vi "Autonomous Independent.vi"() -> ()   [LabVIEW 2016]
doc: "This VI is called when autonomous begins, and will automatically be terminated when autonomous ends. You can carry out timed or sensor driven robot movement independently without needing to return to the caller."
uses:
  <vilib>/Rock Robotics/WPI/Solenoid/WPI_SolenoidValue.ctl
  <vilib>/Rock Robotics/WPI/Utilities/WPI_GetSetVariantRefNum.vi
  <vilib>/addons/control/pid/pid.llb/PID (DBL).vi
  <vilib>/Rock Robotics/Network Tables/NT Write Number.vi
  <vilib>/Rock Robotics/WPI/RobotDrive/WPI_RobotDriveMecanumDrive_Cartesian.vi
  <vilib>/Rock Robotics/WPI/Solenoid/WPI_SolenoidSetEnum.vi
  <vilib>/addons/control/pid/NI_PID_pid.lvlib
panel:
  in  "PID gains 8":T1={"proportional gain (Kc)"=0.055, "integral time (Ti, min)"=0.0, "derivative time (Td, min)"=0.0} {"derivative time (Td, min)" format="%.3f"; "integral time (Ti, min)" format="%.3f"; "proportional gain (Kc)" format="%.3f"}
  out "Gauge 11":dbl(knob) scale=-180.0..180.0
  out "Gryo angle 11":dbl
  out "to motor 8":dbl
  in  "PID gains 12":T1={"proportional gain (Kc)"=0.055, "integral time (Ti, min)"=0.0, "derivative time (Td, min)"=0.0} {"derivative time (Td, min)" format="%.3f"; "integral time (Ti, min)" format="%.3f"; "proportional gain (Kc)" format="%.3f"}
  out "Gauge 15":dbl(knob) scale=-180.0..180.0
  out "Gryo angle 15":dbl
  out "to motor 12":dbl
  in  "PID gains 6":T1={"proportional gain (Kc)"=0.057, "integral time (Ti, min)"=0.0, "derivative time (Td, min)"=0.0} {"derivative time (Td, min)" format="%.3f"; "integral time (Ti, min)" format="%.3f"; "proportional gain (Kc)" format="%.3f"}
  out "Gauge 9":dbl(knob) scale=-180.0..180.0
  out "Gryo angle 9":dbl
  out "to motor 6":dbl
  in  "PID gains 7":T1={"proportional gain (Kc)"=0.055, "integral time (Ti, min)"=0.0, "derivative time (Td, min)"=0.0} {"derivative time (Td, min)" format="%.3f"; "integral time (Ti, min)" format="%.3f"; "proportional gain (Kc)" format="%.3f"}
  out "Gauge 10":dbl(knob) scale=-180.0..180.0
  out "Gryo angle 10":dbl
  out "to motor 7":dbl
  in  "PID gains 16":T1={"proportional gain (Kc)"=0.057, "integral time (Ti, min)"=0.0, "derivative time (Td, min)"=0.0} {"derivative time (Td, min)" format="%.3f"; "integral time (Ti, min)" format="%.3f"; "proportional gain (Kc)" format="%.3f"}
  out "Gauge 19":dbl(knob) scale=-180.0..180.0
  out "Gryo angle 19":dbl
  out "to motor 16":dbl
  in  "PID gains 19":T1={"proportional gain (Kc)"=0.057, "integral time (Ti, min)"=0.0, "derivative time (Td, min)"=0.0} {"derivative time (Td, min)" format="%.3f"; "integral time (Ti, min)" format="%.3f"; "proportional gain (Kc)" format="%.3f"}
  out "Gauge 26":dbl(knob) scale=-180.0..180.0
  out "Gryo angle 26":dbl
  out "to motor 23":dbl
  in  "PID gains 21":T1={"proportional gain (Kc)"=0.057, "integral time (Ti, min)"=0.0, "derivative time (Td, min)"=0.0} {"derivative time (Td, min)" format="%.3f"; "integral time (Ti, min)" format="%.3f"; "proportional gain (Kc)" format="%.3f"}
  out "Gauge 28":dbl(knob) scale=-180.0..180.0
  out "Gryo angle 28":dbl
  out "to motor 25":dbl
  in  "PID gains 48":T1={"proportional gain (Kc)"=0.057, "integral time (Ti, min)"=0.0, "derivative time (Td, min)"=0.0} {"derivative time (Td, min)" format="%.3f"; "integral time (Ti, min)" format="%.3f"; "proportional gain (Kc)" format="%.3f"}
  out "Gauge 55":dbl(knob) scale=-180.0..180.0
  out "Gryo angle 55":dbl
  out "to motor 52":dbl
  in  "PID gains 47":T1={"proportional gain (Kc)"=0.057, "integral time (Ti, min)"=0.0, "derivative time (Td, min)"=0.0} {"derivative time (Td, min)" format="%.3f"; "integral time (Ti, min)" format="%.3f"; "proportional gain (Kc)" format="%.3f"}
  out "Gauge 54":dbl(knob) scale=-180.0..180.0
  out "Gryo angle 54":dbl
  out "to motor 51":dbl
  in  "PID gains 46":T1={"proportional gain (Kc)"=0.057, "integral time (Ti, min)"=0.0, "derivative time (Td, min)"=0.0} {"derivative time (Td, min)" format="%.3f"; "integral time (Ti, min)" format="%.3f"; "proportional gain (Kc)" format="%.3f"}
  out "Gauge 53":dbl(knob) scale=-180.0..180.0
  out "Gryo angle 53":dbl
  out "to motor 50":dbl
  in  "PID gains 45":T1={"proportional gain (Kc)"=0.057, "integral time (Ti, min)"=0.0, "derivative time (Td, min)"=0.0} {"derivative time (Td, min)" format="%.3f"; "integral time (Ti, min)" format="%.3f"; "proportional gain (Kc)" format="%.3f"}
  out "Gauge 52":dbl(knob) scale=-180.0..180.0
  out "Gryo angle 52":dbl
  out "to motor 49":dbl
  in  "PID gains 44":T1={"proportional gain (Kc)"=0.057, "integral time (Ti, min)"=0.0, "derivative time (Td, min)"=0.0} {"derivative time (Td, min)" format="%.3f"; "integral time (Ti, min)" format="%.3f"; "proportional gain (Kc)" format="%.3f"}
  out "Gauge 51":dbl(knob) scale=-180.0..180.0
  out "Gryo angle 51":dbl
  out "to motor 48":dbl
  in  "PID gains 43":T1={"proportional gain (Kc)"=0.057, "integral time (Ti, min)"=0.0, "derivative time (Td, min)"=0.0} {"derivative time (Td, min)" format="%.3f"; "integral time (Ti, min)" format="%.3f"; "proportional gain (Kc)" format="%.3f"}
  out "Gauge 50":dbl(knob) scale=-180.0..180.0
  out "Gryo angle 50":dbl
  out "to motor 47":dbl
  in  "PID gains 42":T1={"proportional gain (Kc)"=0.057, "integral time (Ti, min)"=0.0, "derivative time (Td, min)"=0.0} {"derivative time (Td, min)" format="%.3f"; "integral time (Ti, min)" format="%.3f"; "proportional gain (Kc)" format="%.3f"}
  out "Gauge 49":dbl(knob) scale=-180.0..180.0
  out "Gryo angle 49":dbl
  out "to motor 46":dbl
  in  "PID gains 29":T1={"proportional gain (Kc)"=0.057, "integral time (Ti, min)"=0.0, "derivative time (Td, min)"=0.0} {"derivative time (Td, min)" format="%.3f"; "integral time (Ti, min)" format="%.3f"; "proportional gain (Kc)" format="%.3f"}
  out "Gauge 36":dbl(knob) scale=-180.0..180.0
  out "Gryo angle 36":dbl
  out "to motor 33":dbl
  in  "PID gains 36":T1={"proportional gain (Kc)"=0.057, "integral time (Ti, min)"=0.0, "derivative time (Td, min)"=0.0} {"derivative time (Td, min)" format="%.3f"; "integral time (Ti, min)" format="%.3f"; "proportional gain (Kc)" format="%.3f"}
  out "Gauge 43":dbl(knob) scale=-180.0..180.0
  out "Gryo angle 43":dbl
  out "to motor 40":dbl
  in  "PID gains 37":T1={"proportional gain (Kc)"=0.057, "integral time (Ti, min)"=0.0, "derivative time (Td, min)"=0.0} {"derivative time (Td, min)" format="%.3f"; "integral time (Ti, min)" format="%.3f"; "proportional gain (Kc)" format="%.3f"}
  out "Gauge 44":dbl(knob) scale=-180.0..180.0
  out "Gryo angle 44":dbl
  out "to motor 41":dbl
  in  "PID gains 38":T1={"proportional gain (Kc)"=0.057, "integral time (Ti, min)"=0.0, "derivative time (Td, min)"=0.0} {"derivative time (Td, min)" format="%.3f"; "integral time (Ti, min)" format="%.3f"; "proportional gain (Kc)" format="%.3f"}
  out "Gauge 45":dbl(knob) scale=-180.0..180.0
  out "Gryo angle 45":dbl
  out "to motor 42":dbl
  in  "PID gains 39":T1={"proportional gain (Kc)"=0.057, "integral time (Ti, min)"=0.0, "derivative time (Td, min)"=0.0} {"derivative time (Td, min)" format="%.3f"; "integral time (Ti, min)" format="%.3f"; "proportional gain (Kc)" format="%.3f"}
  out "Gauge 46":dbl(knob) scale=-180.0..180.0
  out "Gryo angle 46":dbl
  out "to motor 43":dbl
  in  "PID gains 40":T1={"proportional gain (Kc)"=0.057, "integral time (Ti, min)"=0.0, "derivative time (Td, min)"=0.0} {"derivative time (Td, min)" format="%.3f"; "integral time (Ti, min)" format="%.3f"; "proportional gain (Kc)" format="%.3f"}
  out "Gauge 47":dbl(knob) scale=-180.0..180.0
  out "Gryo angle 47":dbl
  out "to motor 44":dbl
  in  "PID gains 41":T1={"proportional gain (Kc)"=0.057, "integral time (Ti, min)"=0.0, "derivative time (Td, min)"=0.0} {"derivative time (Td, min)" format="%.3f"; "integral time (Ti, min)" format="%.3f"; "proportional gain (Kc)" format="%.3f"}
  out "Gauge 48":dbl(knob) scale=-180.0..180.0
  out "Gryo angle 48":dbl
  out "to motor 45":dbl
  in  "PID gains 28":T1={"proportional gain (Kc)"=0.057, "integral time (Ti, min)"=0.0, "derivative time (Td, min)"=0.0} {"derivative time (Td, min)" format="%.3f"; "integral time (Ti, min)" format="%.3f"; "proportional gain (Kc)" format="%.3f"}
  out "Gauge 35":dbl(knob) scale=-180.0..180.0
  out "Gryo angle 35":dbl
  out "to motor 32":dbl
  in  "PID gains 30":T1={"proportional gain (Kc)"=0.057, "integral time (Ti, min)"=0.0, "derivative time (Td, min)"=0.0} {"derivative time (Td, min)" format="%.3f"; "integral time (Ti, min)" format="%.3f"; "proportional gain (Kc)" format="%.3f"}
  out "Gauge 37":dbl(knob) scale=-180.0..180.0
  out "Gryo angle 37":dbl
  out "to motor 34":dbl
  in  "PID gains 31":T1={"proportional gain (Kc)"=0.057, "integral time (Ti, min)"=0.0, "derivative time (Td, min)"=0.0} {"derivative time (Td, min)" format="%.3f"; "integral time (Ti, min)" format="%.3f"; "proportional gain (Kc)" format="%.3f"}
  out "Gauge 38":dbl(knob) scale=-180.0..180.0
  out "Gryo angle 38":dbl
  out "to motor 35":dbl
  in  "PID gains 32":T1={"proportional gain (Kc)"=0.057, "integral time (Ti, min)"=0.0, "derivative time (Td, min)"=0.0} {"derivative time (Td, min)" format="%.3f"; "integral time (Ti, min)" format="%.3f"; "proportional gain (Kc)" format="%.3f"}
  out "Gauge 39":dbl(knob) scale=-180.0..180.0
  out "Gryo angle 39":dbl
  out "to motor 36":dbl
  in  "PID gains 33":T1={"proportional gain (Kc)"=0.057, "integral time (Ti, min)"=0.0, "derivative time (Td, min)"=0.0} {"derivative time (Td, min)" format="%.3f"; "integral time (Ti, min)" format="%.3f"; "proportional gain (Kc)" format="%.3f"}
  out "Gauge 40":dbl(knob) scale=-180.0..180.0
  out "Gryo angle 40":dbl
  out "to motor 37":dbl
  in  "PID gains 34":T1={"proportional gain (Kc)"=0.057, "integral time (Ti, min)"=0.0, "derivative time (Td, min)"=0.0} {"derivative time (Td, min)" format="%.3f"; "integral time (Ti, min)" format="%.3f"; "proportional gain (Kc)" format="%.3f"}
  out "Gauge 41":dbl(knob) scale=-180.0..180.0
  out "Gryo angle 41":dbl
  out "to motor 38":dbl
  in  "PID gains 35":T1={"proportional gain (Kc)"=0.057, "integral time (Ti, min)"=0.0, "derivative time (Td, min)"=0.0} {"derivative time (Td, min)" format="%.3f"; "integral time (Ti, min)" format="%.3f"; "proportional gain (Kc)" format="%.3f"}
  out "Gauge 42":dbl(knob) scale=-180.0..180.0
  out "Gryo angle 42":dbl
  out "to motor 39":dbl
  in  "PID gains 23":T1={"proportional gain (Kc)"=0.057, "integral time (Ti, min)"=0.0, "derivative time (Td, min)"=0.0} {"derivative time (Td, min)" format="%.3f"; "integral time (Ti, min)" format="%.3f"; "proportional gain (Kc)" format="%.3f"}
  out "Gauge 30":dbl(knob) scale=-180.0..180.0
  out "Gryo angle 30":dbl
  out "to motor 27":dbl
  in  "PID gains 20":T1={"proportional gain (Kc)"=0.057, "integral time (Ti, min)"=0.0, "derivative time (Td, min)"=0.0} {"derivative time (Td, min)" format="%.3f"; "integral time (Ti, min)" format="%.3f"; "proportional gain (Kc)" format="%.3f"}
  out "Gauge 27":dbl(knob) scale=-180.0..180.0
  out "Gryo angle 27":dbl
  out "to motor 24":dbl
  in  "PID gains 22":T1={"proportional gain (Kc)"=0.057, "integral time (Ti, min)"=0.0, "derivative time (Td, min)"=0.0} {"derivative time (Td, min)" format="%.3f"; "integral time (Ti, min)" format="%.3f"; "proportional gain (Kc)" format="%.3f"}
  out "Gauge 29":dbl(knob) scale=-180.0..180.0
  out "Gryo angle 29":dbl
  out "to motor 26":dbl
  in  "PID gains 24":T1={"proportional gain (Kc)"=0.057, "integral time (Ti, min)"=0.0, "derivative time (Td, min)"=0.0} {"derivative time (Td, min)" format="%.3f"; "integral time (Ti, min)" format="%.3f"; "proportional gain (Kc)" format="%.3f"}
  out "Gauge 31":dbl(knob) scale=-180.0..180.0
  out "Gryo angle 31":dbl
  out "to motor 28":dbl
  in  "PID gains 25":T1={"proportional gain (Kc)"=0.057, "integral time (Ti, min)"=0.0, "derivative time (Td, min)"=0.0} {"derivative time (Td, min)" format="%.3f"; "integral time (Ti, min)" format="%.3f"; "proportional gain (Kc)" format="%.3f"}
  out "Gauge 32":dbl(knob) scale=-180.0..180.0
  out "Gryo angle 32":dbl
  out "to motor 29":dbl
  in  "PID gains 26":T1={"proportional gain (Kc)"=0.057, "integral time (Ti, min)"=0.0, "derivative time (Td, min)"=0.0} {"derivative time (Td, min)" format="%.3f"; "integral time (Ti, min)" format="%.3f"; "proportional gain (Kc)" format="%.3f"}
  out "Gauge 33":dbl(knob) scale=-180.0..180.0
  out "Gryo angle 33":dbl
  out "to motor 30":dbl
  in  "PID gains 15":T1={"proportional gain (Kc)"=0.057, "integral time (Ti, min)"=0.0, "derivative time (Td, min)"=0.0} {"derivative time (Td, min)" format="%.3f"; "integral time (Ti, min)" format="%.3f"; "proportional gain (Kc)" format="%.3f"}
  out "Gauge 18":dbl(knob) scale=-180.0..180.0
  out "Gryo angle 18":dbl
  out "to motor 15":dbl
  in  "PID gains 14":T1={"proportional gain (Kc)"=0.055, "integral time (Ti, min)"=0.0, "derivative time (Td, min)"=0.0} {"derivative time (Td, min)" format="%.3f"; "integral time (Ti, min)" format="%.3f"; "proportional gain (Kc)" format="%.3f"}
  out "Gauge 17":dbl(knob) scale=-180.0..180.0
  out "Gryo angle 17":dbl
  out "to motor 14":dbl
  out "Gauge 21":dbl(knob) scale=-180.0..180.0
  out "Gryo angle 21":dbl
  out "to motor 18":dbl
  out "Gauge 22":dbl(knob) scale=-180.0..180.0
  out "Gryo angle 22":dbl
  out "to motor 19":dbl
  in  "PID gains 17":T1={"proportional gain (Kc)"=0.055, "integral time (Ti, min)"=0.0, "derivative time (Td, min)"=0.0} {"derivative time (Td, min)" format="%.3f"; "integral time (Ti, min)" format="%.3f"; "proportional gain (Kc)" format="%.3f"}
  out "Gauge 20":dbl(knob) scale=-180.0..180.0
  out "Gryo angle 20":dbl
  out "to motor 17":dbl
  in  "PID gains 18":T1={"proportional gain (Kc)"=0.055, "integral time (Ti, min)"=0.0, "derivative time (Td, min)"=0.0} {"derivative time (Td, min)" format="%.3f"; "integral time (Ti, min)" format="%.3f"; "proportional gain (Kc)" format="%.3f"}
  out "Gauge 24":dbl(knob) scale=-180.0..180.0
  out "Gryo angle 24":dbl
  out "to motor 21":dbl
  out "Gauge 25":dbl(knob) scale=-180.0..180.0
  out "Gryo angle 25":dbl
  out "to motor 22":dbl
  out "Gauge 23":dbl(knob) scale=-180.0..180.0
  out "Gryo angle 23":dbl
  out "to motor 20":dbl
  # "Be sure to right-click and choose Data Operations>>Make Current Value default if you want to save the array values with the VI"
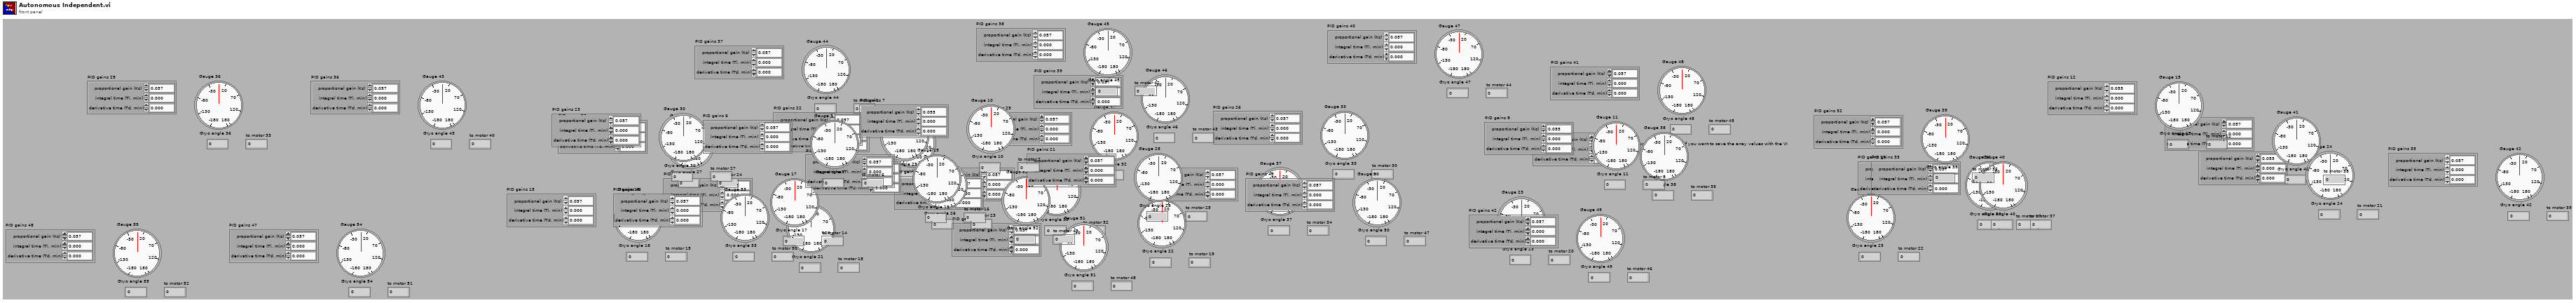
[diagram p1: front panel]
types:
  T1 = cluster{"proportional gain (Kc)":dbl, "integral time (Ti, min)":dbl, "derivative time (Td, min)":dbl}
  T2 = enum16{"None", "Tank", "Drive strait", "Square", "Place Gear Center", "Place Gear Left", "Place Gear Right ", "Place Gear Right/ Shoot"}
  T3 = typedef "WPI_JoystickDevRef.ctl" = cluster{"Device":T4}
  T4 = typedef "WPI_JoystickDeviceEnum.ctl" = enum16{"USB 0", "USB 1", "USB 2", "USB 3", "USB 4", "USB 5"}
  T5 = typedef "WPI_SolenoidDevRef.ctl" = cluster{"DevStatus":errorcluster, "Pneumatics Control Module":u8, "Forward Solenoid Channel":T6, "Reverse Solenoid Channel":T6}
  T6 = typedef "WPI_SolenoidChannel.ctl" = enum8{"Solenoid 0", "Solenoid 1", "Solenoid 2", "Solenoid 3", "Solenoid 4", "Solenoid 5", "Solenoid 6", "Solenoid 7", "Invalid"}
  T7 = typedef "WPI_RobotDriveDevRef.ctl" = cluster{"DevStatus":errorcluster, "Motors[]":T8[], "Square Inputs":bool, "Max Output":dbl}
  T8 = typedef "WPI_MotorControlDeviceRef.ctl" = cluster{"DeviceStatus":errorcluster, "Type":T9, "PWM":cluster{"PWM Channel":T10, "DeadBand":T11}, "CAN":cluster{"Device Number":u8, "SetOutput VI Ref":variant, "GetOutput VI Ref":variant, "Enable VI Ref":variant, "Disable VI Ref":variant, "Data":variant}, "Invert":bool}
  T9 = typedef "WPI_MotorControlType.ctl" = enum16{"PWM", "CAN"}
  T10 = typedef "FPGA_DIOPWMChannel.ctl" = enum8{"PWM 0", "PWM 1", "PWM 2", "PWM 3", "PWM 4", "PWM 5", "PWM 6", "PWM 7", "PWM 8", "PWM 9", "PWM MXP 0", "PWM MXP 1", "PWM MXP 2", "PWM MXP 3", "PWM MXP 4", "PWM MXP 5", "PWM MXP 6", "PWM MXP 7", "PWM MXP 8", "PWM MXP 9", "Invalid"}
  T11 = typedef "WPI_PWMDeadband.ctl" = cluster{"Name":string, "maxPositivePwm":i32, "minPositivePwm":i32, "centerPwm":i32, "maxNegativePwm":i32, "minNegativePwm":i32, "angularRange":u16}
  T12 = typedef "WPI_SolenoidValue.ctl" = enum16{"Off", "On", "Forward", "Reverse"}
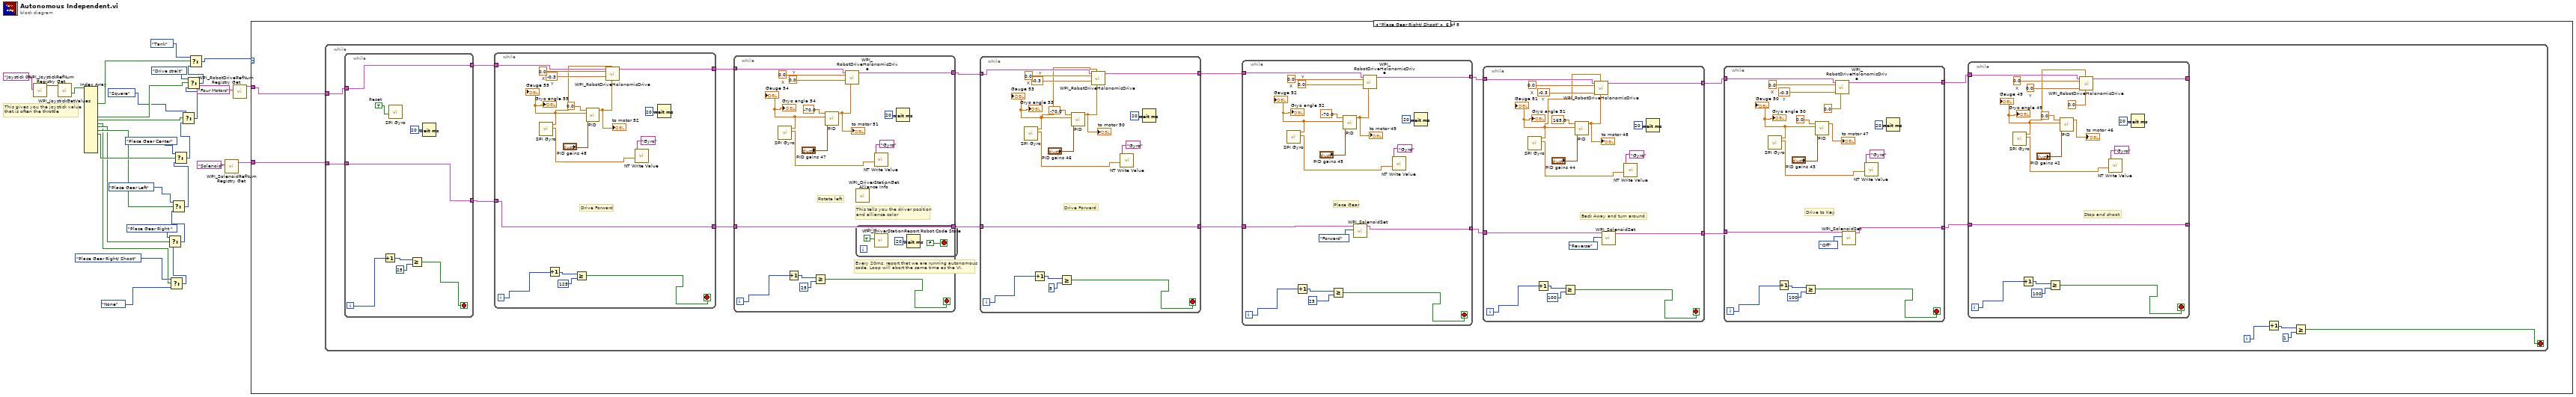
[diagram p0: block diagram]
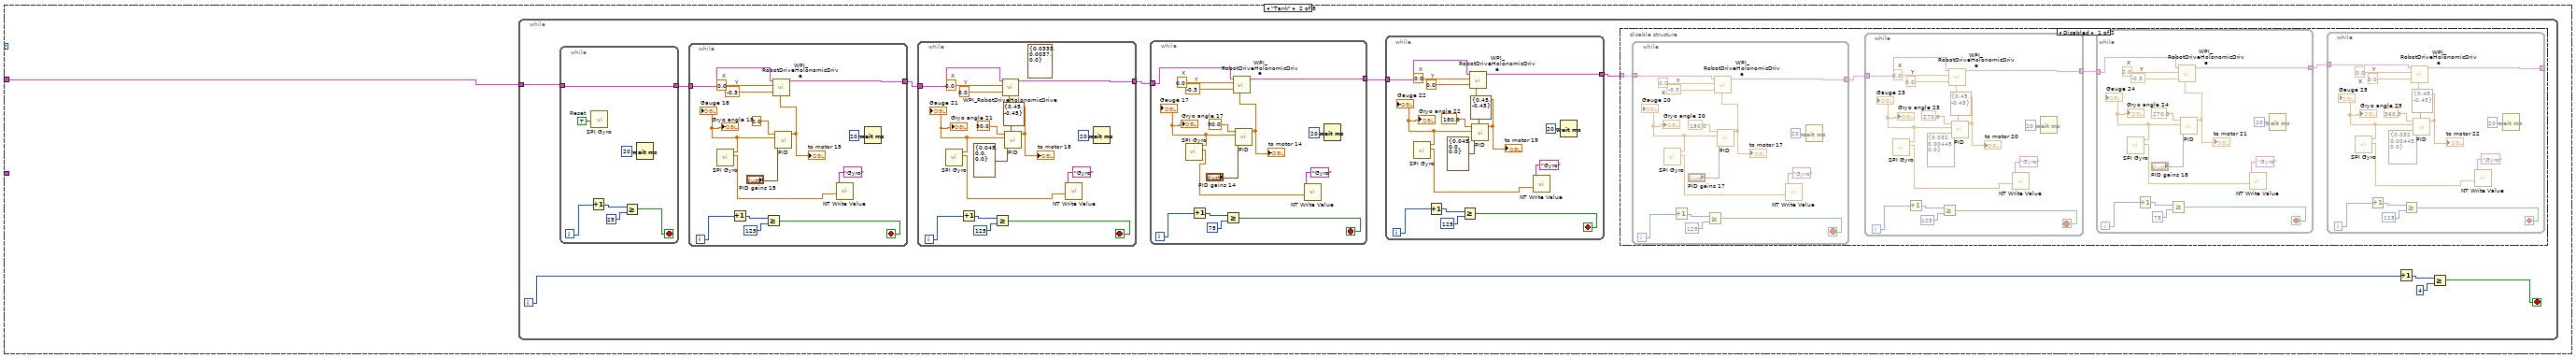
[diagram p3: hidden frame]
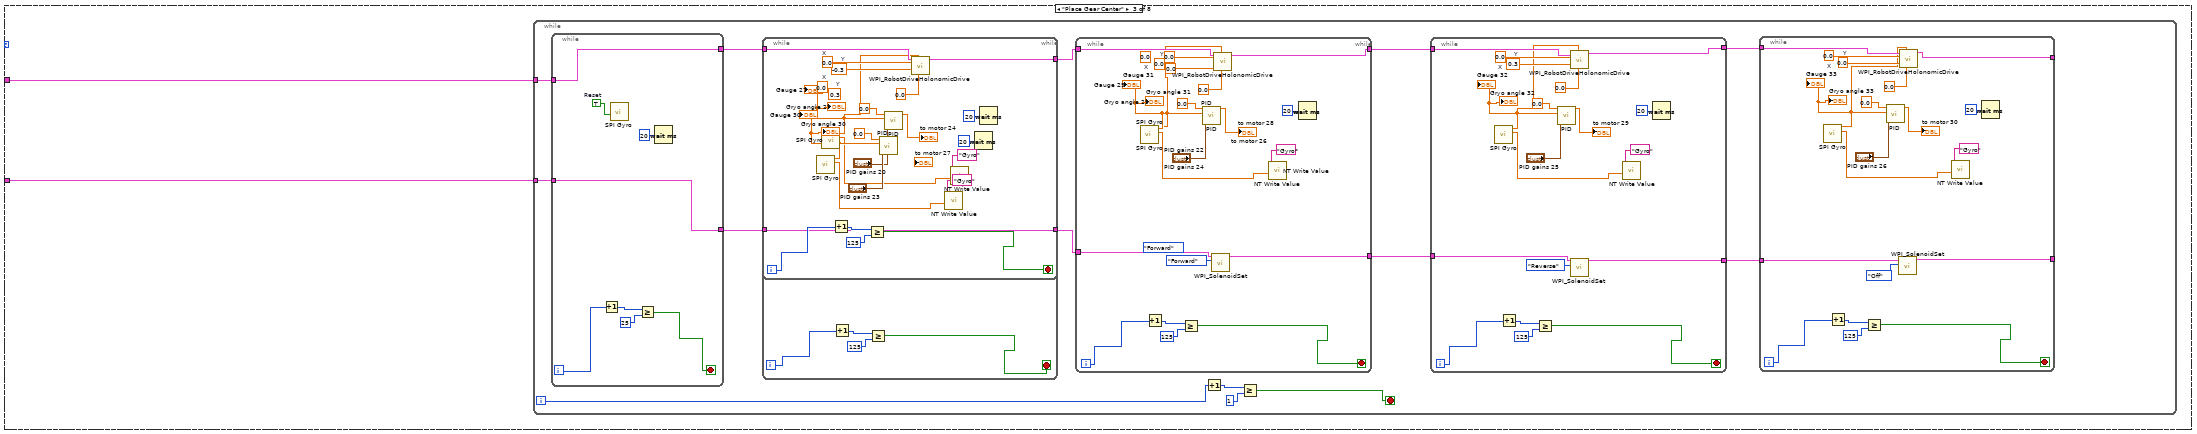
[diagram p5: hidden frame]
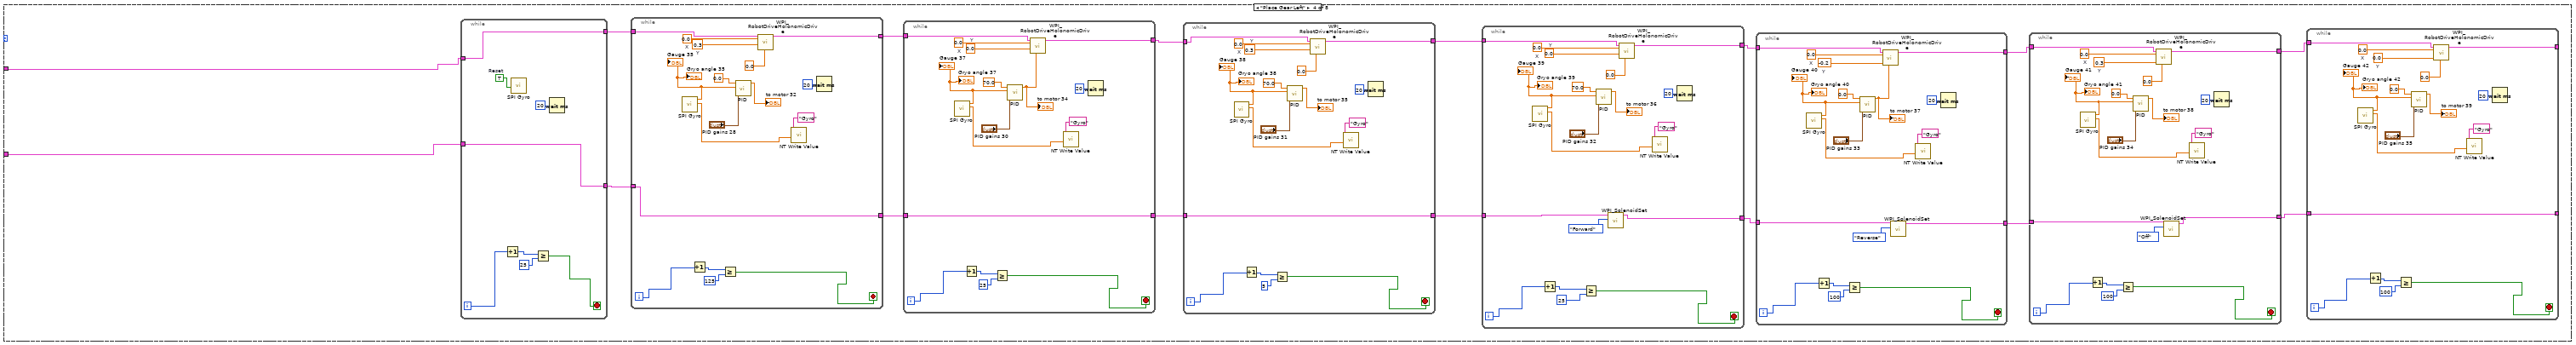
[diagram p6: hidden frame]
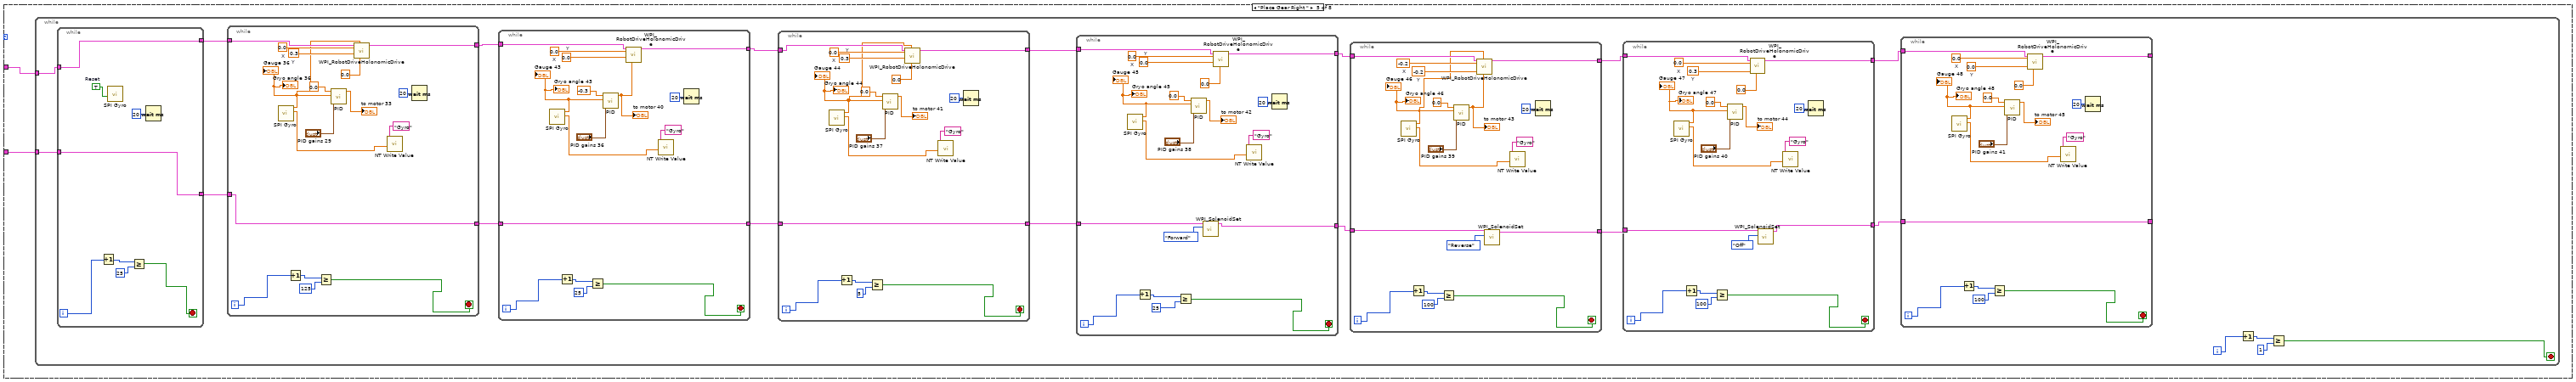
[diagram p7: hidden frame]
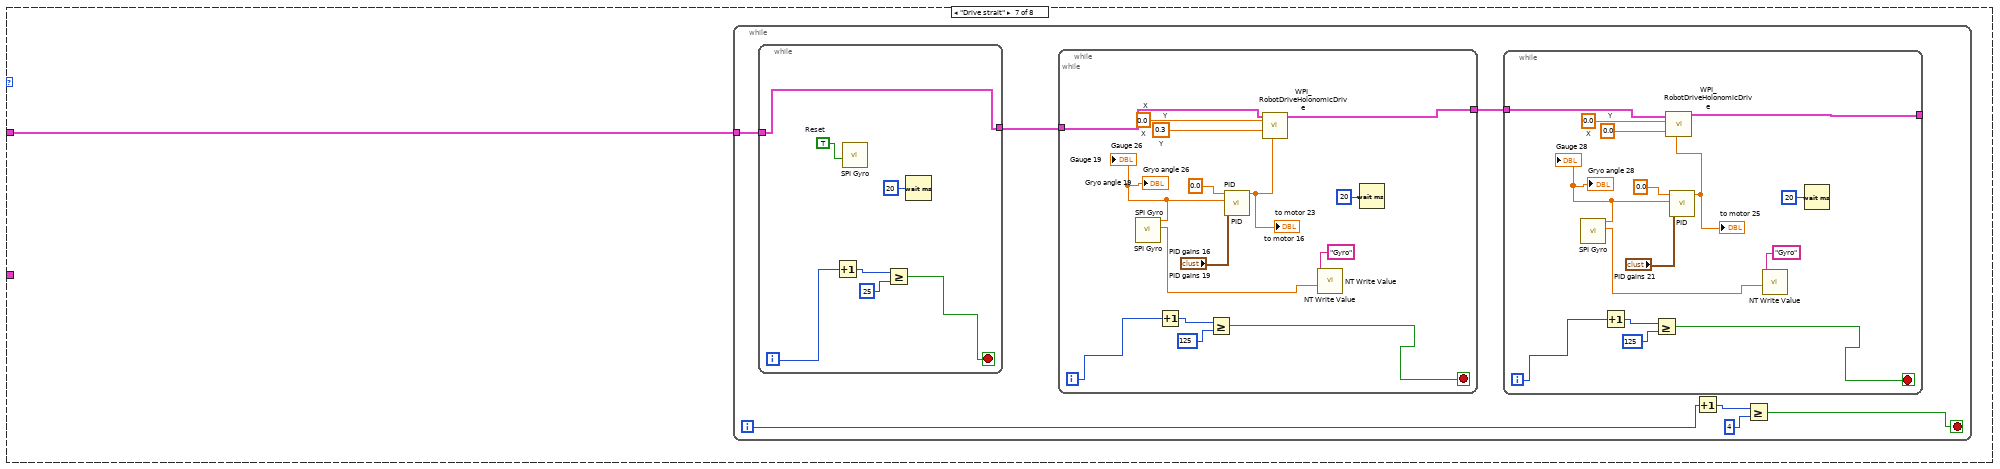
[diagram p8: hidden frame]
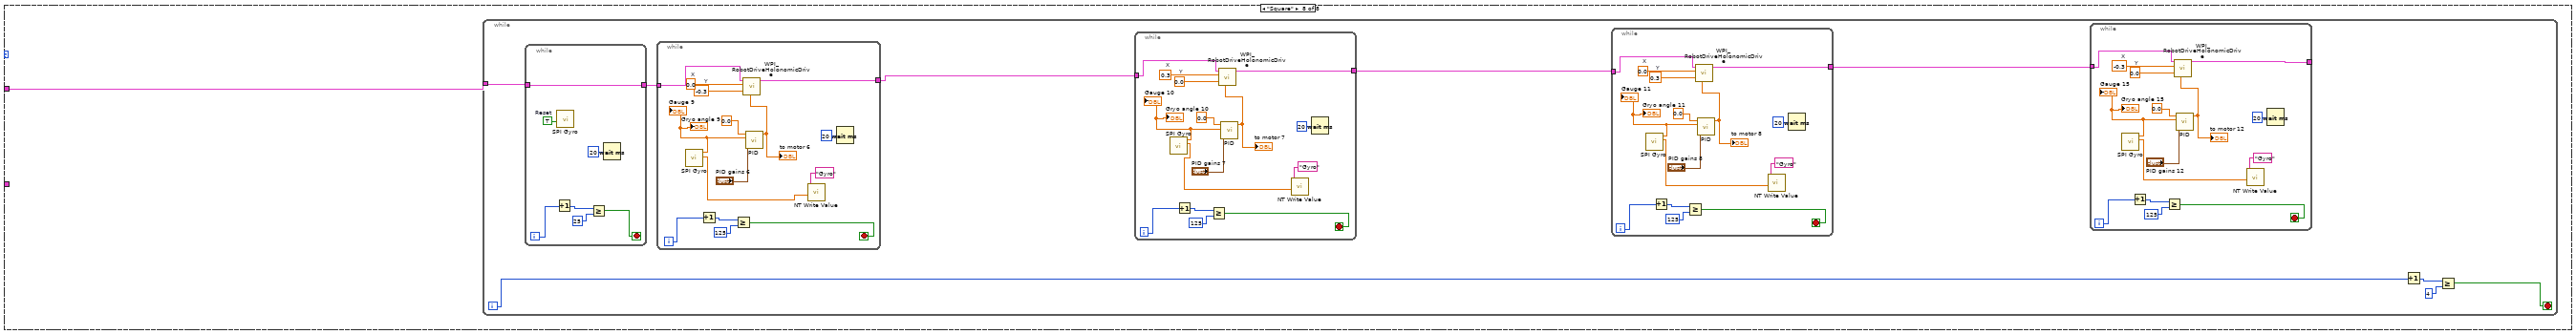
[diagram p9: hidden frame]
diagram:
  # "This gives you the joystick value\nthat is often the throttle"
  # "Every 20ms, report that we are running autonomous\ncode. Loop will abort the same time as the VI."
  # "This tells you the driver position\nand alliance color"
  n1 = call <vilib>:"WPI_JoystickRefNum Registry Get.vi"("refnum name"="Joystick 0") -> ("JoystickDevRef"=w29:T3)  [unwired: 1 in, 9 out]
  n2 = call <vilib>:"WPI_JoystickGetValues.vi"("JoystickDevRef"=w29) -> ("Buttons"=w28:bool[])  [unwired: 6 in, 4 out]
  n3 = Index Array(array=w28) -> (element #4=w27:bool, element #7=w25:bool, element #8=w22:bool, element #9=w4:bool, element #10=w12:bool, element #11=w16:bool, element #12=w17:bool)  [unwired: 17 in, 10 out]
  n4 = Select(t=T2."Place Gear Right/ Shoot", s=w4, f=T2."None") -> (s? t:f=w2:T2)
  n5 = Select(t=T2."Place Gear Right ", s=w12, f=w2) -> (s? t:f=w11:T2)
  n6 = Select(t=T2."Place Gear Left", s=w16, f=w11) -> (s? t:f=w15:T2)
  n7 = Select(t=T2."Place Gear Center", s=w17, f=w15) -> (s? t:f=w20:T2)
  n8 = Select(t=T2."Square", s=w22, f=w20) -> (s? t:f=w21:T2)
  n9 = Select(t=T2."Drive strait", s=w25, f=w21) -> (s? t:f=w26:T2)
  n10 = Select(t=T2."Tank", s=w27, f=w26) -> (s? t:f=w14:T2)
  n11 = call <vilib>:"WPI_SolenoidRefNum Registry Get.vi"("refnum name"="Solenoid") -> ("SolenoidDevRef"=w18:T5)  [unwired: 9 in, 1 out]
  n12 = call <vilib>:"WPI_RobotDriveRefNum Registry Get.vi"("refnum name"="Four Motors") -> ("RobotDriveDevRef"=w23:T7)  [unwired: 9 in, 1 out]
  n13 = case shown="\"Place Gear Right/ Shoot\"" w14 {
    tunnel: w23 -> [_ w30 w177 w310 w442 w596 w745 w800]
    tunnel: w18 -> [_ _ w176 w309 w443 w595 _ _]
    frame "None", Default {
    }
    frame "Tank" {
      n14 = while {
        tunnel: w30 -> [w39]
        i -> [w35]
        stop <- w36 stop-if-true
        n15 = while {
          tunnel: [w175] -> w40
          tunnel: w39 -> [w175]
          i -> [w171]
          stop <- w172 stop-if-true
          w169 = TRUE  # Reset
          n16 = Increment(x=w171) -> (x+1=w174:i32)
          n17 = call "SPI Gyro.vi"("Reset"=w169) -> ()  [unwired: 8 in, 3 out]
          n18 = Greater Or Equal?(x=w174, y=25) -> (x >= y?=w172:bool)
          n19 = Wait (ms)(milliseconds to wait=u32 20) -> ()  [unwired: 1 out]
        }
        n20 = while {
          tunnel: [w168] -> w34
          tunnel: w40 -> [w157]
          i -> [w166]
          stop <- w163 stop-if-true
          w161 = -0.3  # Y
          w162 = 0.0  # X
          n21 = call "SPI Gyro.vi"() -> ("Angle"=w154:dbl, "Raw"=w155:dbl)  [unwired: 9 in, 1 out]
          "Gauge 18" <- w155
          "Gryo angle 18" <- w155
          n22 = Increment(x=w166) -> (x+1=w165:i32)
          n23 = Greater Or Equal?(x=w165, y=125) -> (x >= y?=w163:bool)
          n24 = call-poly <vilib>:"PID.vi"("PID gains"="PID gains 15", "process variable"=w155, "setpoint"=0.0) -> ("output"=w158:dbl)  [unwired: 7 in, 1 out]
          "to motor 15" <- w158
          n25 = call-poly <vilib>:"WPI_RobotDriveHolonomicDrive.vi"("Rotation"=w158, "Y"=w161, "X"=w162, "RobotDriveDevRef"=w157) -> ("RobotDriveDevRef"=w168:T7)  [unwired: 5 in, 2 out]
          n26 = call-poly <vilib>:"NT Write Value.vi"("Numeric"=w154, "Name"="Gyro") -> ()  [unwired: 9 in, 1 out]
          n27 = Wait (ms)(milliseconds to wait=u32 20) -> ()  [unwired: 1 out]
        }
        n28 = while {
          tunnel: [w138] -> w33
          tunnel: w34 -> [w128]
          i -> [w136]
          stop <- w133 stop-if-true
          (unwired) T1 {"proportional gain (Kc)"=0.0335, "integral time (Ti, min)"=0.0037, "derivative time (Td, min)"=0.0} ("PID gains")
          w131 = 0.0  # Y
          w132 = 0.0  # X
          n29 = call "SPI Gyro.vi"() -> ("Angle"=w125:dbl, "Raw"=w126:dbl)  [unwired: 9 in, 1 out]
          "Gauge 21" <- w126
          "Gryo angle 21" <- w126
          n30 = Increment(x=w136) -> (x+1=w135:i32)
          n31 = Greater Or Equal?(x=w135, y=125) -> (x >= y?=w133:bool)
          n32 = call-poly <vilib>:"PID.vi"("output range"=cluster{"output high":dbl, "output low":dbl} {"output high"=0.45, "output low"=-0.45}, "PID gains"=T1 {"proportional gain (Kc)"=0.045, "integral time (Ti, min)"=0.0, "derivative time (Td, min)"=0.0}, "process variable"=w126, "setpoint"=90.0) -> ("output"=w129:dbl)  [unwired: 6 in, 1 out]
          "to motor 18" <- w129
          n33 = call-poly <vilib>:"WPI_RobotDriveHolonomicDrive.vi"("Rotation"=w129, "Y"=w131, "X"=w132, "RobotDriveDevRef"=w128) -> ("RobotDriveDevRef"=w138:T7)  [unwired: 5 in, 2 out]
          n34 = call-poly <vilib>:"NT Write Value.vi"("Numeric"=w125, "Name"="Gyro") -> ()  [unwired: 9 in, 1 out]
          n35 = Wait (ms)(milliseconds to wait=u32 20) -> ()  [unwired: 1 out]
        }
        n36 = while {
          tunnel: [w153] -> w32
          tunnel: w33 -> [w142]
          i -> [w151]
          stop <- w148 stop-if-true
          w146 = -0.3  # Y
          w147 = 0.0  # X
          n37 = call "SPI Gyro.vi"() -> ("Angle"=w139:dbl, "Raw"=w140:dbl)  [unwired: 9 in, 1 out]
          "Gauge 17" <- w140
          "Gryo angle 17" <- w140
          n38 = Increment(x=w151) -> (x+1=w150:i32)
          n39 = Greater Or Equal?(x=w150, y=75) -> (x >= y?=w148:bool)
          n40 = call-poly <vilib>:"PID.vi"("PID gains"="PID gains 14", "process variable"=w140, "setpoint"=90.0) -> ("output"=w143:dbl)  [unwired: 7 in, 1 out]
          "to motor 14" <- w143
          n41 = call-poly <vilib>:"WPI_RobotDriveHolonomicDrive.vi"("Rotation"=w143, "Y"=w146, "X"=w147, "RobotDriveDevRef"=w142) -> ("RobotDriveDevRef"=w153:T7)  [unwired: 5 in, 2 out]
          n42 = call-poly <vilib>:"NT Write Value.vi"("Numeric"=w139, "Name"="Gyro") -> ()  [unwired: 9 in, 1 out]
          n43 = Wait (ms)(milliseconds to wait=u32 20) -> ()  [unwired: 1 out]
        }
        n44 = while {
          tunnel: [w122] -> w31
          tunnel: w32 -> [w112]
          i -> [w120]
          stop <- w117 stop-if-true
          w115 = 0.0  # Y
          w116 = 0.0  # X
          n45 = call "SPI Gyro.vi"() -> ("Angle"=w109:dbl, "Raw"=w110:dbl)  [unwired: 9 in, 1 out]
          "Gauge 22" <- w110
          "Gryo angle 22" <- w110
          n46 = Increment(x=w120) -> (x+1=w119:i32)
          n47 = Greater Or Equal?(x=w119, y=125) -> (x >= y?=w117:bool)
          n48 = call-poly <vilib>:"PID.vi"("output range"=cluster{"output high":dbl, "output low":dbl} {"output high"=0.45, "output low"=-0.45}, "PID gains"=T1 {"proportional gain (Kc)"=0.045, "integral time (Ti, min)"=0.0, "derivative time (Td, min)"=0.0}, "process variable"=w110, "setpoint"=180.0) -> ("output"=w113:dbl)  [unwired: 6 in, 1 out]
          "to motor 19" <- w113
          n49 = call-poly <vilib>:"WPI_RobotDriveHolonomicDrive.vi"("Rotation"=w113, "Y"=w115, "X"=w116, "RobotDriveDevRef"=w112) -> ("RobotDriveDevRef"=w122:T7)  [unwired: 5 in, 2 out]
          n50 = call-poly <vilib>:"NT Write Value.vi"("Numeric"=w109, "Name"="Gyro") -> ()  [unwired: 9 in, 1 out]
          n51 = Wait (ms)(milliseconds to wait=u32 20) -> ()  [unwired: 1 out]
        }
        n52 = disable-structure shown="Disabled" {
          disable-tunnel: w31 -> [w43 _]
          frame Disabled {
            n53 = while {
              tunnel: [w106] -> w42
              tunnel: w43 -> [w92]
              i -> [w104]
              stop <- w101 stop-if-true
              w99 = -0.3  # Y
              w100 = 0.0  # X
              n54 = call "SPI Gyro.vi"() -> ("Angle"=w93:dbl, "Raw"=w94:dbl)  [unwired: 9 in, 1 out]
              "Gauge 20" <- w94
              "Gryo angle 20" <- w94
              n55 = Increment(x=w104) -> (x+1=w103:i32)
              n56 = Greater Or Equal?(x=w103, y=125) -> (x >= y?=w101:bool)
              n57 = call-poly <vilib>:"PID.vi"("PID gains"="PID gains 17", "process variable"=w94, "setpoint"=180.0) -> ("output"=w96:dbl)  [unwired: 7 in, 1 out]
              "to motor 17" <- w96
              n58 = call-poly <vilib>:"WPI_RobotDriveHolonomicDrive.vi"("Rotation"=w96, "Y"=w99, "X"=w100, "RobotDriveDevRef"=w92) -> ("RobotDriveDevRef"=w106:T7)  [unwired: 5 in, 2 out]
              n59 = call-poly <vilib>:"NT Write Value.vi"("Numeric"=w93, "Name"="Gyro") -> ()  [unwired: 9 in, 1 out]
              n60 = Wait (ms)(milliseconds to wait=u32 20) -> ()  [unwired: 1 out]
            }
            n61 = while {
              tunnel: [w60] -> w44
              tunnel: w42 -> [w50]
              i -> [w58]
              stop <- w55 stop-if-true
              w53 = 0.0  # Y
              w54 = 0.0  # X
              n62 = call "SPI Gyro.vi"() -> ("Angle"=w47:dbl, "Raw"=w48:dbl)  [unwired: 9 in, 1 out]
              "Gauge 23" <- w48
              "Gryo angle 23" <- w48
              n63 = Increment(x=w58) -> (x+1=w57:i32)
              n64 = Greater Or Equal?(x=w57, y=125) -> (x >= y?=w55:bool)
              n65 = call-poly <vilib>:"PID.vi"("output range"=cluster{"output high":dbl, "output low":dbl} {"output high"=0.45, "output low"=-0.45}, "PID gains"=T1 {"proportional gain (Kc)"=0.032, "integral time (Ti, min)"=0.00445, "derivative time (Td, min)"=0.0}, "process variable"=w48, "setpoint"=270.0) -> ("output"=w51:dbl)  [unwired: 6 in, 1 out]
              "to motor 20" <- w51
              n66 = call-poly <vilib>:"WPI_RobotDriveHolonomicDrive.vi"("Rotation"=w51, "Y"=w53, "X"=w54, "RobotDriveDevRef"=w50) -> ("RobotDriveDevRef"=w60:T7)  [unwired: 5 in, 2 out]
              n67 = call-poly <vilib>:"NT Write Value.vi"("Numeric"=w47, "Name"="Gyro") -> ()  [unwired: 9 in, 1 out]
              n68 = Wait (ms)(milliseconds to wait=u32 20) -> ()  [unwired: 1 out]
            }
            n69 = while {
              tunnel: [w91] -> w41
              tunnel: w44 -> [w80]
              i -> [w89]
              stop <- w86 stop-if-true
              w84 = -0.3  # Y
              w85 = 0.0  # X
              n70 = call "SPI Gyro.vi"() -> ("Angle"=w77:dbl, "Raw"=w78:dbl)  [unwired: 9 in, 1 out]
              "Gauge 24" <- w78
              "Gryo angle 24" <- w78
              n71 = Increment(x=w89) -> (x+1=w88:i32)
              n72 = Greater Or Equal?(x=w88, y=75) -> (x >= y?=w86:bool)
              n73 = call-poly <vilib>:"PID.vi"("PID gains"="PID gains 18", "process variable"=w78, "setpoint"=270.0) -> ("output"=w81:dbl)  [unwired: 7 in, 1 out]
              "to motor 21" <- w81
              n74 = call-poly <vilib>:"WPI_RobotDriveHolonomicDrive.vi"("Rotation"=w81, "Y"=w84, "X"=w85, "RobotDriveDevRef"=w80) -> ("RobotDriveDevRef"=w91:T7)  [unwired: 5 in, 2 out]
              n75 = call-poly <vilib>:"NT Write Value.vi"("Numeric"=w77, "Name"="Gyro") -> ()  [unwired: 9 in, 1 out]
              n76 = Wait (ms)(milliseconds to wait=u32 20) -> ()  [unwired: 1 out]
            }
            n77 = while {
              tunnel: [w76] -> _
              tunnel: w41 -> [w61]
              i -> [w74]
              stop <- w71 stop-if-true
              w69 = 0.0  # Y
              w70 = 0.0  # X
              n78 = call "SPI Gyro.vi"() -> ("Angle"=w64:dbl, "Raw"=w65:dbl)  [unwired: 9 in, 1 out]
              "Gauge 25" <- w65
              "Gryo angle 25" <- w65
              n79 = Increment(x=w74) -> (x+1=w73:i32)
              n80 = Greater Or Equal?(x=w73, y=125) -> (x >= y?=w71:bool)
              n81 = call-poly <vilib>:"PID.vi"("output range"=cluster{"output high":dbl, "output low":dbl} {"output high"=0.45, "output low"=-0.45}, "PID gains"=T1 {"proportional gain (Kc)"=0.032, "integral time (Ti, min)"=0.00445, "derivative time (Td, min)"=0.0}, "process variable"=w65, "setpoint"=360.0) -> ("output"=w67:dbl)  [unwired: 6 in, 1 out]
              "to motor 22" <- w67
              n82 = call-poly <vilib>:"WPI_RobotDriveHolonomicDrive.vi"("Rotation"=w67, "Y"=w69, "X"=w70, "RobotDriveDevRef"=w61) -> ("RobotDriveDevRef"=w76:T7)  [unwired: 5 in, 2 out]
              n83 = call-poly <vilib>:"NT Write Value.vi"("Numeric"=w64, "Name"="Gyro") -> ()  [unwired: 9 in, 1 out]
              n84 = Wait (ms)(milliseconds to wait=u32 20) -> ()  [unwired: 1 out]
            }
          }
          frame Enabled {
          }
        }
        n85 = Increment(x=w35) -> (x+1=w37:i32)
        n86 = Greater Or Equal?(x=w37, y=4) -> (x >= y?=w36:bool)
      }
    }
    frame "Place Gear Center" {
      n87 = while {
        tunnel: w177 -> [w186]
        tunnel: w176 -> [w181]
        i -> [w188]
        stop <- w189 stop-if-true
        n88 = while {
          tunnel: [w278] -> w187
          tunnel: w186 -> [w278]
          tunnel: [w277] -> w182
          tunnel: w181 -> [w277]
          i -> [w280]
          stop <- w279 stop-if-true
          w281 = TRUE  # Reset
          n89 = Increment(x=w280) -> (x+1=w284:i32)
          n90 = call "SPI Gyro.vi"("Reset"=w281) -> ()  [unwired: 8 in, 3 out]
          n91 = Greater Or Equal?(x=w284, y=25) -> (x >= y?=w279:bool)
          n92 = Wait (ms)(milliseconds to wait=u32 20) -> ()  [unwired: 1 out]
        }
        n93 = while {
          tunnel: w187 -> [w264]
          tunnel: [w263] -> w185
          tunnel: [w262] -> w183
          tunnel: w182 -> [w262]
          i -> [w269]
          stop <- w268 stop-if-true
          w267 = -0.3  # Y
          w266 = 0.0  # X
          n94 = call "SPI Gyro.vi"() -> ("Angle"=w270:dbl, "Raw"=w260:dbl)  [unwired: 9 in, 1 out]
          "Gauge 27" <- w260
          "Gryo angle 27" <- w260
          n95 = Increment(x=w269) -> (x+1=w275:i32)
          n96 = Greater Or Equal?(x=w275, y=125) -> (x >= y?=w268:bool)
          n97 = call-poly <vilib>:"PID.vi"("PID gains"="PID gains 20", "process variable"=w260, "setpoint"=0.0) -> ("output"=→"to motor 24":dbl)  [unwired: 7 in, 1 out]
          n98 = call-poly <vilib>:"WPI_RobotDriveHolonomicDrive.vi"("Rotation"=0.0, "Gyro Angle"=w260, "Y"=w267, "X"=w266, "RobotDriveDevRef"=w264) -> ("RobotDriveDevRef"=w263:T7)  [unwired: 4 in, 2 out]
          n99 = call-poly <vilib>:"NT Write Value.vi"("Numeric"=w270, "Name"="Gyro") -> ()  [unwired: 9 in, 1 out]
          n100 = Wait (ms)(milliseconds to wait=u32 20) -> ()  [unwired: 1 out]
        }
        n101 = while {
          i -> [w286]
          stop <- w285 stop-if-true
          (unwired) 0.3  # Y
          (unwired) 0.0  # X
          n102 = call "SPI Gyro.vi"() -> ("Angle"=w287:dbl, "Raw"=w288:dbl)  [unwired: 9 in, 1 out]
          "Gauge 30" <- w288
          "Gryo angle 30" <- w288
          n103 = Increment(x=w286) -> (x+1=w293:i32)
          n104 = Greater Or Equal?(x=w293, y=125) -> (x >= y?=w285:bool)
          n105 = call-poly <vilib>:"PID.vi"("PID gains"="PID gains 23", "process variable"=w288, "setpoint"=0.0) -> ()  [unwired: 7 in, 2 out]
          n106 = call-poly <vilib>:"NT Write Value.vi"("Numeric"=w287, "Name"="Gyro") -> ()  [unwired: 9 in, 1 out]
          n107 = Wait (ms)(milliseconds to wait=u32 20) -> ()  [unwired: 1 out]
        }
        n108 = while {
          tunnel: w185 -> [w236]
          tunnel: w183 -> [w238]
          tunnel: [w237] -> w180
          tunnel: [w235] -> w178
          i -> [w241]
          stop <- w240 stop-if-true
          n109 = call "SPI Gyro.vi"() -> ("Angle"=w242:dbl, "Raw"=w230:dbl)  [unwired: 9 in, 1 out]
          "Gauge 31" <- w230
          "Gryo angle 31" <- w230
          n110 = Increment(x=w241) -> (x+1=w247:i32)
          n111 = Greater Or Equal?(x=w247, y=125) -> (x >= y?=w240:bool)
          n112 = call-poly <vilib>:"PID.vi"("PID gains"="PID gains 24", "process variable"=w230, "setpoint"=0.0) -> ("output"=→"to motor 28":dbl)  [unwired: 7 in, 1 out]
          n113 = call-poly <vilib>:"WPI_SolenoidSet.vi"("Value"=WPI_SolenoidValue."Forward", "SolenoidDevRef"=w238) -> ("SolenoidDevRef"=w237:T5)  [unwired: 8 in, 1 out]
          n114 = call-poly <vilib>:"WPI_RobotDriveHolonomicDrive.vi"("Rotation"=0.0, "Gyro Angle"=w230, "Y"=0.0, "X"=0.0, "RobotDriveDevRef"=w236) -> ("RobotDriveDevRef"=w235:T7)  [unwired: 4 in, 2 out]
          n115 = call-poly <vilib>:"NT Write Value.vi"("Numeric"=w242, "Name"="Gyro") -> ()  [unwired: 9 in, 1 out]
          n116 = Wait (ms)(milliseconds to wait=u32 20) -> ()  [unwired: 1 out]
        }
        n117 = while {
          i -> [w250]
          stop <- w249 stop-if-true
          (unwired) WPI_SolenoidValue."Forward" ("Value")
          (unwired) 0.0  # Y
          (unwired) 0.0  # X
          n118 = call "SPI Gyro.vi"() -> ("Angle"=w251:dbl, "Raw"=w252:dbl)  [unwired: 9 in, 1 out]
          "Gauge 29" <- w252
          "Gryo angle 29" <- w252
          n119 = Increment(x=w250) -> (x+1=w258:i32)
          n120 = Greater Or Equal?(x=w258, y=125) -> (x >= y?=w249:bool)
          n121 = call-poly <vilib>:"PID.vi"("PID gains"="PID gains 22", "process variable"=w252, "setpoint"=0.0) -> ("output"=→"to motor 26":dbl)  [unwired: 7 in, 1 out]
          n122 = call-poly <vilib>:"NT Write Value.vi"("Numeric"=w251, "Name"="Gyro") -> ()  [unwired: 9 in, 1 out]
          n123 = Wait (ms)(milliseconds to wait=u32 20) -> ()  [unwired: 1 out]
        }
        n124 = Increment(x=w188) -> (x+1=w190:i32)
        n125 = Greater Or Equal?(x=w190, y=1) -> (x >= y?=w189:bool)
        n126 = while {
          tunnel: [w216] -> w184
          tunnel: w180 -> [w215]
          tunnel: [w214] -> w179
          tunnel: w178 -> [w213]
          i -> [w219]
          stop <- w218 stop-if-true
          w225 = 0.3  # Y
          w226 = 0.0  # X
          n127 = call "SPI Gyro.vi"() -> ("Angle"=w220:dbl, "Raw"=w211:dbl)  [unwired: 9 in, 1 out]
          "Gauge 32" <- w211
          "Gryo angle 32" <- w211
          n128 = Increment(x=w219) -> (x+1=w228:i32)
          n129 = Greater Or Equal?(x=w228, y=125) -> (x >= y?=w218:bool)
          n130 = call-poly <vilib>:"PID.vi"("PID gains"="PID gains 25", "process variable"=w211, "setpoint"=0.0) -> ("output"=→"to motor 29":dbl)  [unwired: 7 in, 1 out]
          n131 = call-poly <vilib>:"WPI_SolenoidSet.vi"("Value"=WPI_SolenoidValue."Reverse", "SolenoidDevRef"=w215) -> ("SolenoidDevRef"=w214:T5)  [unwired: 8 in, 1 out]
          n132 = call-poly <vilib>:"WPI_RobotDriveHolonomicDrive.vi"("Rotation"=0.0, "Gyro Angle"=w211, "Y"=w225, "X"=w226, "RobotDriveDevRef"=w213) -> ("RobotDriveDevRef"=w216:T7)  [unwired: 4 in, 2 out]
          n133 = call-poly <vilib>:"NT Write Value.vi"("Numeric"=w220, "Name"="Gyro") -> ()  [unwired: 9 in, 1 out]
          n134 = Wait (ms)(milliseconds to wait=u32 20) -> ()  [unwired: 1 out]
        }
        n135 = while {
          tunnel: w184 -> [w197]
          tunnel: [w196] -> _
          tunnel: w179 -> [w195]
          tunnel: [w194] -> _
          i -> [w200]
          stop <- w199 stop-if-true
          w206 = 0.0  # Y
          w207 = 0.0  # X
          n136 = call "SPI Gyro.vi"() -> ("Angle"=w201:dbl, "Raw"=w192:dbl)  [unwired: 9 in, 1 out]
          "Gauge 33" <- w192
          "Gryo angle 33" <- w192
          n137 = Increment(x=w200) -> (x+1=w209:i32)
          n138 = Greater Or Equal?(x=w209, y=125) -> (x >= y?=w199:bool)
          n139 = call-poly <vilib>:"PID.vi"("PID gains"="PID gains 26", "process variable"=w192, "setpoint"=0.0) -> ("output"=→"to motor 30":dbl)  [unwired: 7 in, 1 out]
          n140 = call-poly <vilib>:"WPI_SolenoidSet.vi"("Value"=WPI_SolenoidValue."Off", "SolenoidDevRef"=w195) -> ("SolenoidDevRef"=w194:T5)  [unwired: 8 in, 1 out]
          n141 = call-poly <vilib>:"WPI_RobotDriveHolonomicDrive.vi"("Rotation"=0.0, "Gyro Angle"=w192, "Y"=w206, "X"=w207, "RobotDriveDevRef"=w197) -> ("RobotDriveDevRef"=w196:T7)  [unwired: 4 in, 2 out]
          n142 = call-poly <vilib>:"NT Write Value.vi"("Numeric"=w201, "Name"="Gyro") -> ()  [unwired: 9 in, 1 out]
          n143 = Wait (ms)(milliseconds to wait=u32 20) -> ()  [unwired: 1 out]
        }
      }
    }
    frame "Place Gear Left" {
      n144 = while {
        tunnel: [w418] -> w308
        tunnel: w310 -> [w418]
        tunnel: [w417] -> w304
        tunnel: w309 -> [w417]
        i -> [w420]
        stop <- w419 stop-if-true
        w421 = TRUE  # Reset
        n145 = Increment(x=w420) -> (x+1=w424:i32)
        n146 = call "SPI Gyro.vi"("Reset"=w421) -> ()  [unwired: 8 in, 3 out]
        n147 = Greater Or Equal?(x=w424, y=25) -> (x >= y?=w419:bool)
        n148 = Wait (ms)(milliseconds to wait=u32 20) -> ()  [unwired: 1 out]
      }
      n149 = while {
        tunnel: [w428] -> w307
        tunnel: w308 -> [w426]
        tunnel: w304 -> [w425]
        tunnel: [w425] -> w303
        i -> [w433]
        stop <- w432 stop-if-true
        w431 = 0.3  # Y
        w430 = 0.0  # X
        n150 = call "SPI Gyro.vi"() -> ("Angle"=w434:dbl, "Raw"=w435:dbl)  [unwired: 9 in, 1 out]
        "Gauge 35" <- w435
        "Gryo angle 35" <- w435
        n151 = Increment(x=w433) -> (x+1=w440:i32)
        n152 = Greater Or Equal?(x=w440, y=125) -> (x >= y?=w432:bool)
        n153 = call-poly <vilib>:"PID.vi"("PID gains"="PID gains 28", "process variable"=w435, "setpoint"=0.0) -> ("output"=→"to motor 32":dbl)  [unwired: 7 in, 1 out]
        n154 = call-poly <vilib>:"WPI_RobotDriveHolonomicDrive.vi"("Rotation"=0.0, "Y"=w431, "X"=w430, "RobotDriveDevRef"=w426) -> ("RobotDriveDevRef"=w428:T7)  [unwired: 5 in, 2 out]
        n155 = call-poly <vilib>:"NT Write Value.vi"("Numeric"=w434, "Name"="Gyro") -> ()  [unwired: 9 in, 1 out]
        n156 = Wait (ms)(milliseconds to wait=u32 20) -> ()  [unwired: 1 out]
      }
      n157 = while {
        tunnel: [w404] -> w306
        tunnel: w307 -> [w403]
        tunnel: w303 -> [w401]
        tunnel: [w401] -> w302
        i -> [w408]
        stop <- w407 stop-if-true
        w406 = 0.0  # Y
        w405 = 0.0  # X
        n158 = call "SPI Gyro.vi"() -> ("Angle"=w409:dbl, "Raw"=w410:dbl)  [unwired: 9 in, 1 out]
        "Gauge 37" <- w410
        "Gryo angle 37" <- w410
        n159 = Increment(x=w408) -> (x+1=w415:i32)
        n160 = Greater Or Equal?(x=w415, y=25) -> (x >= y?=w407:bool)
        n161 = call-poly <vilib>:"PID.vi"("PID gains"="PID gains 30", "process variable"=w410, "setpoint"=70.0) -> ("output"=w402:dbl)  [unwired: 7 in, 1 out]
        "to motor 34" <- w402
        n162 = call-poly <vilib>:"WPI_RobotDriveHolonomicDrive.vi"("Rotation"=w402, "Y"=w406, "X"=w405, "RobotDriveDevRef"=w403) -> ("RobotDriveDevRef"=w404:T7)  [unwired: 5 in, 2 out]
        n163 = call-poly <vilib>:"NT Write Value.vi"("Numeric"=w409, "Name"="Gyro") -> ()  [unwired: 9 in, 1 out]
        n164 = Wait (ms)(milliseconds to wait=u32 20) -> ()  [unwired: 1 out]
      }
      n165 = while {
        tunnel: [w388] -> w305
        tunnel: w306 -> [w386]
        tunnel: w302 -> [w384]
        tunnel: [w384] -> w301
        i -> [w392]
        stop <- w391 stop-if-true
        w390 = 0.3  # Y
        w389 = 0.0  # X
        n166 = call "SPI Gyro.vi"() -> ("Angle"=w393:dbl, "Raw"=w394:dbl)  [unwired: 9 in, 1 out]
        "Gauge 38" <- w394
        "Gryo angle 38" <- w394
        n167 = Increment(x=w392) -> (x+1=w399:i32)
        n168 = Greater Or Equal?(x=w399, y=5) -> (x >= y?=w391:bool)
        n169 = call-poly <vilib>:"PID.vi"("PID gains"="PID gains 31", "process variable"=w394, "setpoint"=70.0) -> ("output"=→"to motor 35":dbl)  [unwired: 7 in, 1 out]
        n170 = call-poly <vilib>:"WPI_RobotDriveHolonomicDrive.vi"("Rotation"=0.0, "Y"=w390, "X"=w389, "RobotDriveDevRef"=w386) -> ("RobotDriveDevRef"=w388:T7)  [unwired: 5 in, 2 out]
        n171 = call-poly <vilib>:"NT Write Value.vi"("Numeric"=w393, "Name"="Gyro") -> ()  [unwired: 9 in, 1 out]
        n172 = Wait (ms)(milliseconds to wait=u32 20) -> ()  [unwired: 1 out]
      }
      n173 = while {
        tunnel: [w371] -> w299
        tunnel: w305 -> [w370]
        tunnel: w301 -> [w366]
        tunnel: [w365] -> w300
        i -> [w375]
        stop <- w374 stop-if-true
        w373 = 0.0  # Y
        w372 = 0.0  # X
        n174 = call "SPI Gyro.vi"() -> ("Angle"=w376:dbl, "Raw"=w377:dbl)  [unwired: 9 in, 1 out]
        "Gauge 39" <- w377
        "Gryo angle 39" <- w377
        n175 = Increment(x=w375) -> (x+1=w382:i32)
        n176 = Greater Or Equal?(x=w382, y=25) -> (x >= y?=w374:bool)
        n177 = call-poly <vilib>:"PID.vi"("PID gains"="PID gains 32", "process variable"=w377, "setpoint"=70.0) -> ("output"=→"to motor 36":dbl)  [unwired: 7 in, 1 out]
        n178 = call-poly <vilib>:"WPI_SolenoidSet.vi"("Value"=WPI_SolenoidValue."Forward", "SolenoidDevRef"=w366) -> ("SolenoidDevRef"=w365:T5)  [unwired: 8 in, 1 out]
        n179 = call-poly <vilib>:"WPI_RobotDriveHolonomicDrive.vi"("Rotation"=0.0, "Y"=w373, "X"=w372, "RobotDriveDevRef"=w370) -> ("RobotDriveDevRef"=w371:T7)  [unwired: 5 in, 2 out]
        n180 = call-poly <vilib>:"NT Write Value.vi"("Numeric"=w376, "Name"="Gyro") -> ()  [unwired: 9 in, 1 out]
        n181 = Wait (ms)(milliseconds to wait=u32 20) -> ()  [unwired: 1 out]
      }
      n182 = while {
        tunnel: [w352] -> w297
        tunnel: w299 -> [w351]
        tunnel: w300 -> [w349]
        tunnel: [w347] -> w298
        i -> [w356]
        stop <- w355 stop-if-true
        w354 = -0.2  # Y
        w353 = 0.0  # X
        n183 = call "SPI Gyro.vi"() -> ("Angle"=w357:dbl, "Raw"=w358:dbl)  [unwired: 9 in, 1 out]
        "Gauge 40" <- w358
        "Gryo angle 40" <- w358
        n184 = Increment(x=w356) -> (x+1=w363:i32)
        n185 = Greater Or Equal?(x=w363, y=100) -> (x >= y?=w355:bool)
        n186 = call-poly <vilib>:"PID.vi"("PID gains"="PID gains 33", "process variable"=w358, "setpoint"=0.0) -> ("output"=w348:dbl)  [unwired: 7 in, 1 out]
        "to motor 37" <- w348
        n187 = call-poly <vilib>:"WPI_RobotDriveHolonomicDrive.vi"("Rotation"=w348, "Y"=w354, "X"=w353, "RobotDriveDevRef"=w351) -> ("RobotDriveDevRef"=w352:T7)  [unwired: 5 in, 2 out]
        n188 = call-poly <vilib>:"WPI_SolenoidSet.vi"("Value"=WPI_SolenoidValue."Reverse", "SolenoidDevRef"=w349) -> ("SolenoidDevRef"=w347:T5)  [unwired: 8 in, 1 out]
        n189 = call-poly <vilib>:"NT Write Value.vi"("Numeric"=w357, "Name"="Gyro") -> ()  [unwired: 9 in, 1 out]
        n190 = Wait (ms)(milliseconds to wait=u32 20) -> ()  [unwired: 1 out]
      }
      n191 = while {
        tunnel: [w334] -> w296
        tunnel: w297 -> [w333]
        tunnel: w298 -> [w331]
        tunnel: [w328] -> w295
        i -> [w338]
        stop <- w337 stop-if-true
        w336 = 0.3  # Y
        w335 = 0.0  # X
        n192 = call "SPI Gyro.vi"() -> ("Angle"=w339:dbl, "Raw"=w340:dbl)  [unwired: 9 in, 1 out]
        "Gauge 41" <- w340
        "Gryo angle 41" <- w340
        n193 = Increment(x=w338) -> (x+1=w345:i32)
        n194 = Greater Or Equal?(x=w345, y=100) -> (x >= y?=w337:bool)
        n195 = call-poly <vilib>:"PID.vi"("PID gains"="PID gains 34", "process variable"=w340, "setpoint"=0.0) -> ("output"=→"to motor 38":dbl)  [unwired: 7 in, 1 out]
        n196 = call-poly <vilib>:"WPI_RobotDriveHolonomicDrive.vi"("Rotation"=0.0, "Y"=w336, "X"=w335, "RobotDriveDevRef"=w333) -> ("RobotDriveDevRef"=w334:T7)  [unwired: 5 in, 2 out]
        n197 = call-poly <vilib>:"WPI_SolenoidSet.vi"("Value"=WPI_SolenoidValue."Off", "SolenoidDevRef"=w331) -> ("SolenoidDevRef"=w328:T5)  [unwired: 8 in, 1 out]
        n198 = call-poly <vilib>:"NT Write Value.vi"("Numeric"=w339, "Name"="Gyro") -> ()  [unwired: 9 in, 1 out]
        n199 = Wait (ms)(milliseconds to wait=u32 20) -> ()  [unwired: 1 out]
      }
      n200 = while {
        tunnel: [w315] -> _
        tunnel: w296 -> [w314]
        tunnel: [w311] -> _
        tunnel: w295 -> [w311]
        i -> [w319]
        stop <- w318 stop-if-true
        w317 = 0.0  # Y
        w316 = 0.0  # X
        n201 = call "SPI Gyro.vi"() -> ("Angle"=w320:dbl, "Raw"=w321:dbl)  [unwired: 9 in, 1 out]
        "Gauge 42" <- w321
        "Gryo angle 42" <- w321
        n202 = Increment(x=w319) -> (x+1=w326:i32)
        n203 = Greater Or Equal?(x=w326, y=100) -> (x >= y?=w318:bool)
        n204 = call-poly <vilib>:"PID.vi"("PID gains"="PID gains 35", "process variable"=w321, "setpoint"=0.0) -> ("output"=→"to motor 39":dbl)  [unwired: 7 in, 1 out]
        n205 = call-poly <vilib>:"WPI_RobotDriveHolonomicDrive.vi"("Rotation"=0.0, "Y"=w317, "X"=w316, "RobotDriveDevRef"=w314) -> ("RobotDriveDevRef"=w315:T7)  [unwired: 5 in, 2 out]
        n206 = call-poly <vilib>:"NT Write Value.vi"("Numeric"=w320, "Name"="Gyro") -> ()  [unwired: 9 in, 1 out]
        n207 = Wait (ms)(milliseconds to wait=u32 20) -> ()  [unwired: 1 out]
      }
    }
    frame "Place Gear Right " {
      n208 = while {
        tunnel: w443 -> [w449]
        tunnel: w442 -> [w448]
        i -> [w444]
        stop <- w445 stop-if-true
        n209 = while {
          tunnel: [w571] -> w450
          tunnel: w448 -> [w571]
          tunnel: [w570] -> w454
          tunnel: w449 -> [w570]
          i -> [w573]
          stop <- w572 stop-if-true
          w574 = TRUE  # Reset
          n210 = Increment(x=w573) -> (x+1=w577:i32)
          n211 = call "SPI Gyro.vi"("Reset"=w574) -> ()  [unwired: 8 in, 3 out]
          n212 = Greater Or Equal?(x=w577, y=25) -> (x >= y?=w572:bool)
          n213 = Wait (ms)(milliseconds to wait=u32 20) -> ()  [unwired: 1 out]
        }
        n214 = while {
          tunnel: [w582] -> w451
          tunnel: w450 -> [w580]
          tunnel: w454 -> [w579]
          tunnel: [w579] -> w455
          i -> [w587]
          stop <- w586 stop-if-true
          w585 = 0.3  # Y
          w584 = 0.0  # X
          n215 = call "SPI Gyro.vi"() -> ("Angle"=w588:dbl, "Raw"=w578:dbl)  [unwired: 9 in, 1 out]
          "Gauge 36" <- w578
          "Gryo angle 36" <- w578
          n216 = Increment(x=w587) -> (x+1=w593:i32)
          n217 = Greater Or Equal?(x=w593, y=125) -> (x >= y?=w586:bool)
          n218 = call-poly <vilib>:"PID.vi"("PID gains"="PID gains 29", "process variable"=w578, "setpoint"=0.0) -> ("output"=→"to motor 33":dbl)  [unwired: 7 in, 1 out]
          n219 = call-poly <vilib>:"WPI_RobotDriveHolonomicDrive.vi"("Rotation"=0.0, "Gyro Angle"=w578, "Y"=w585, "X"=w584, "RobotDriveDevRef"=w580) -> ("RobotDriveDevRef"=w582:T7)  [unwired: 4 in, 2 out]
          n220 = call-poly <vilib>:"NT Write Value.vi"("Numeric"=w588, "Name"="Gyro") -> ()  [unwired: 9 in, 1 out]
          n221 = Wait (ms)(milliseconds to wait=u32 20) -> ()  [unwired: 1 out]
        }
        n222 = while {
          tunnel: [w557] -> w452
          tunnel: w451 -> [w556]
          tunnel: w455 -> [w554]
          tunnel: [w554] -> w456
          i -> [w561]
          stop <- w560 stop-if-true
          w559 = 0.0  # Y
          w558 = 0.0  # X
          n223 = call "SPI Gyro.vi"() -> ("Angle"=w562:dbl, "Raw"=w563:dbl)  [unwired: 9 in, 1 out]
          "Gauge 43" <- w563
          "Gryo angle 43" <- w563
          n224 = Increment(x=w561) -> (x+1=w568:i32)
          n225 = Greater Or Equal?(x=w568, y=25) -> (x >= y?=w560:bool)
          n226 = call-poly <vilib>:"PID.vi"("PID gains"="PID gains 36", "process variable"=w563, "setpoint"=-0.3) -> ("output"=w555:dbl)  [unwired: 7 in, 1 out]
          "to motor 40" <- w555
          n227 = call-poly <vilib>:"WPI_RobotDriveHolonomicDrive.vi"("Rotation"=w555, "Y"=w559, "X"=w558, "RobotDriveDevRef"=w556) -> ("RobotDriveDevRef"=w557:T7)  [unwired: 5 in, 2 out]
          n228 = call-poly <vilib>:"NT Write Value.vi"("Numeric"=w562, "Name"="Gyro") -> ()  [unwired: 9 in, 1 out]
          n229 = Wait (ms)(milliseconds to wait=u32 20) -> ()  [unwired: 1 out]
        }
        n230 = while {
          tunnel: [w542] -> w453
          tunnel: w452 -> [w540]
          tunnel: w456 -> [w538]
          tunnel: [w538] -> w457
          i -> [w546]
          stop <- w545 stop-if-true
          w544 = 0.3  # Y
          w543 = 0.0  # X
          n231 = call "SPI Gyro.vi"() -> ("Angle"=w547:dbl, "Raw"=w537:dbl)  [unwired: 9 in, 1 out]
          "Gauge 44" <- w537
          "Gryo angle 44" <- w537
          n232 = Increment(x=w546) -> (x+1=w552:i32)
          n233 = Greater Or Equal?(x=w552, y=5) -> (x >= y?=w545:bool)
          n234 = call-poly <vilib>:"PID.vi"("PID gains"="PID gains 37", "process variable"=w537, "setpoint"=0.0) -> ("output"=→"to motor 41":dbl)  [unwired: 7 in, 1 out]
          n235 = call-poly <vilib>:"WPI_RobotDriveHolonomicDrive.vi"("Rotation"=0.0, "Gyro Angle"=w537, "Y"=w544, "X"=w543, "RobotDriveDevRef"=w540) -> ("RobotDriveDevRef"=w542:T7)  [unwired: 4 in, 2 out]
          n236 = call-poly <vilib>:"NT Write Value.vi"("Numeric"=w547, "Name"="Gyro") -> ()  [unwired: 9 in, 1 out]
          n237 = Wait (ms)(milliseconds to wait=u32 20) -> ()  [unwired: 1 out]
        }
        n238 = while {
          tunnel: [w524] -> w459
          tunnel: w453 -> [w523]
          tunnel: w457 -> [w519]
          tunnel: [w518] -> w458
          i -> [w528]
          stop <- w527 stop-if-true
          w526 = 0.0  # Y
          w525 = 0.0  # X
          n239 = call "SPI Gyro.vi"() -> ("Angle"=w529:dbl, "Raw"=w530:dbl)  [unwired: 9 in, 1 out]
          "Gauge 45" <- w530
          "Gryo angle 45" <- w530
          n240 = Increment(x=w528) -> (x+1=w535:i32)
          n241 = Greater Or Equal?(x=w535, y=25) -> (x >= y?=w527:bool)
          n242 = call-poly <vilib>:"PID.vi"("PID gains"="PID gains 38", "process variable"=w530, "setpoint"=0.0) -> ("output"=→"to motor 42":dbl)  [unwired: 7 in, 1 out]
          n243 = call-poly <vilib>:"WPI_SolenoidSet.vi"("Value"=WPI_SolenoidValue."Forward", "SolenoidDevRef"=w519) -> ("SolenoidDevRef"=w518:T5)  [unwired: 8 in, 1 out]
          n244 = call-poly <vilib>:"WPI_RobotDriveHolonomicDrive.vi"("Rotation"=0.0, "Y"=w526, "X"=w525, "RobotDriveDevRef"=w523) -> ("RobotDriveDevRef"=w524:T7)  [unwired: 5 in, 2 out]
          n245 = call-poly <vilib>:"NT Write Value.vi"("Numeric"=w529, "Name"="Gyro") -> ()  [unwired: 9 in, 1 out]
          n246 = Wait (ms)(milliseconds to wait=u32 20) -> ()  [unwired: 1 out]
        }
        n247 = while {
          tunnel: [w506] -> w461
          tunnel: w459 -> [w505]
          tunnel: w458 -> [w503]
          tunnel: [w501] -> w460
          i -> [w510]
          stop <- w509 stop-if-true
          w508 = -0.2  # Y
          w507 = -0.2  # X
          n248 = call "SPI Gyro.vi"() -> ("Angle"=w511:dbl, "Raw"=w500:dbl)  [unwired: 9 in, 1 out]
          "Gauge 46" <- w500
          "Gryo angle 46" <- w500
          n249 = Increment(x=w510) -> (x+1=w516:i32)
          n250 = Greater Or Equal?(x=w516, y=100) -> (x >= y?=w509:bool)
          n251 = call-poly <vilib>:"PID.vi"("PID gains"="PID gains 39", "process variable"=w500, "setpoint"=0.0) -> ("output"=w502:dbl)  [unwired: 7 in, 1 out]
          "to motor 43" <- w502
          n252 = call-poly <vilib>:"WPI_RobotDriveHolonomicDrive.vi"("Rotation"=w502, "Gyro Angle"=w500, "Y"=w508, "X"=w507, "RobotDriveDevRef"=w505) -> ("RobotDriveDevRef"=w506:T7)  [unwired: 4 in, 2 out]
          n253 = call-poly <vilib>:"WPI_SolenoidSet.vi"("Value"=WPI_SolenoidValue."Reverse", "SolenoidDevRef"=w503) -> ("SolenoidDevRef"=w501:T5)  [unwired: 8 in, 1 out]
          n254 = call-poly <vilib>:"NT Write Value.vi"("Numeric"=w511, "Name"="Gyro") -> ()  [unwired: 9 in, 1 out]
          n255 = Wait (ms)(milliseconds to wait=u32 20) -> ()  [unwired: 1 out]
        }
        n256 = while {
          tunnel: [w487] -> w462
          tunnel: w461 -> [w486]
          tunnel: w460 -> [w484]
          tunnel: [w481] -> w463
          i -> [w491]
          stop <- w490 stop-if-true
          w489 = 0.3  # Y
          w488 = 0.0  # X
          n257 = call "SPI Gyro.vi"() -> ("Angle"=w492:dbl, "Raw"=w493:dbl)  [unwired: 9 in, 1 out]
          "Gauge 47" <- w493
          "Gryo angle 47" <- w493
          n258 = Increment(x=w491) -> (x+1=w498:i32)
          n259 = Greater Or Equal?(x=w498, y=100) -> (x >= y?=w490:bool)
          n260 = call-poly <vilib>:"PID.vi"("PID gains"="PID gains 40", "process variable"=w493, "setpoint"=0.0) -> ("output"=→"to motor 44":dbl)  [unwired: 7 in, 1 out]
          n261 = call-poly <vilib>:"WPI_RobotDriveHolonomicDrive.vi"("Rotation"=0.0, "Y"=w489, "X"=w488, "RobotDriveDevRef"=w486) -> ("RobotDriveDevRef"=w487:T7)  [unwired: 5 in, 2 out]
          n262 = call-poly <vilib>:"WPI_SolenoidSet.vi"("Value"=WPI_SolenoidValue."Off", "SolenoidDevRef"=w484) -> ("SolenoidDevRef"=w481:T5)  [unwired: 8 in, 1 out]
          n263 = call-poly <vilib>:"NT Write Value.vi"("Numeric"=w492, "Name"="Gyro") -> ()  [unwired: 9 in, 1 out]
          n264 = Wait (ms)(milliseconds to wait=u32 20) -> ()  [unwired: 1 out]
        }
        n265 = while {
          tunnel: [w468] -> _
          tunnel: w462 -> [w467]
          tunnel: [w464] -> _
          tunnel: w463 -> [w464]
          i -> [w472]
          stop <- w471 stop-if-true
          w470 = 0.0  # Y
          w469 = 0.0  # X
          n266 = call "SPI Gyro.vi"() -> ("Angle"=w473:dbl, "Raw"=w474:dbl)  [unwired: 9 in, 1 out]
          "Gauge 48" <- w474
          "Gryo angle 48" <- w474
          n267 = Increment(x=w472) -> (x+1=w479:i32)
          n268 = Greater Or Equal?(x=w479, y=100) -> (x >= y?=w471:bool)
          n269 = call-poly <vilib>:"PID.vi"("PID gains"="PID gains 41", "process variable"=w474, "setpoint"=0.0) -> ("output"=→"to motor 45":dbl)  [unwired: 7 in, 1 out]
          n270 = call-poly <vilib>:"WPI_RobotDriveHolonomicDrive.vi"("Rotation"=0.0, "Y"=w470, "X"=w469, "RobotDriveDevRef"=w467) -> ("RobotDriveDevRef"=w468:T7)  [unwired: 5 in, 2 out]
          n271 = call-poly <vilib>:"NT Write Value.vi"("Numeric"=w473, "Name"="Gyro") -> ()  [unwired: 9 in, 1 out]
          n272 = Wait (ms)(milliseconds to wait=u32 20) -> ()  [unwired: 1 out]
        }
        n273 = Increment(x=w444) -> (x+1=w446:i32)
        n274 = Greater Or Equal?(x=w446, y=1) -> (x >= y?=w445:bool)
      }
    }
    frame "Place Gear Right/ Shoot" {
      n275 = while {
        tunnel: w595 -> [w602]
        tunnel: w596 -> [w601]
        i -> [w597]
        stop <- w598 stop-if-true
        n276 = while {
          tunnel: [w722] -> w603
          tunnel: w601 -> [w722]
          tunnel: [w721] -> w607
          tunnel: w602 -> [w721]
          i -> [w724]
          stop <- w723 stop-if-true
          w725 = TRUE  # Reset
          n277 = Increment(x=w724) -> (x+1=w728:i32)
          n278 = call "SPI Gyro.vi"("Reset"=w725) -> ()  [unwired: 8 in, 3 out]
          n279 = Greater Or Equal?(x=w728, y=25) -> (x >= y?=w723:bool)
          n280 = Wait (ms)(milliseconds to wait=u32 20) -> ()  [unwired: 1 out]
        }
        n281 = while {
          tunnel: [w733] -> w604
          tunnel: w603 -> [w732]
          tunnel: w607 -> [w731]
          tunnel: [w731] -> w608
          i -> [w737]
          stop <- w736 stop-if-true
          w735 = -0.3  # Y
          w734 = 0.0  # X
          # "Drive Forward"
          n282 = call "SPI Gyro.vi"() -> ("Angle"=w738:dbl, "Raw"=w730:dbl)  [unwired: 9 in, 1 out]
          "Gauge 55" <- w730
          "Gryo angle 55" <- w730
          n283 = Increment(x=w737) -> (x+1=w743:i32)
          n284 = Greater Or Equal?(x=w743, y=125) -> (x >= y?=w736:bool)
          n285 = call-poly <vilib>:"PID.vi"("PID gains"="PID gains 48", "process variable"=w730, "setpoint"=0.0) -> ("output"=w729:dbl)  [unwired: 7 in, 1 out]
          "to motor 52" <- w729
          n286 = call-poly <vilib>:"WPI_RobotDriveHolonomicDrive.vi"("Rotation"=w729, "Gyro Angle"=w730, "Y"=w735, "X"=w734, "RobotDriveDevRef"=w732) -> ("RobotDriveDevRef"=w733:T7)  [unwired: 4 in, 2 out]
          n287 = call-poly <vilib>:"NT Write Value.vi"("Numeric"=w738, "Name"="Gyro") -> ()  [unwired: 9 in, 1 out]
          n288 = Wait (ms)(milliseconds to wait=u32 20) -> ()  [unwired: 1 out]
        }
        n289 = while {
          tunnel: [w708] -> w605
          tunnel: w604 -> [w707]
          tunnel: w608 -> [w705]
          tunnel: [w705] -> w609
          i -> [w712]
          stop <- w711 stop-if-true
          w710 = 0.0  # Y
          w709 = 0.0  # X
          # "Rotate left"
          n290 = call "SPI Gyro.vi"() -> ("Angle"=w713:dbl, "Raw"=w714:dbl)  [unwired: 9 in, 1 out]
          "Gauge 54" <- w714
          "Gryo angle 54" <- w714
          n291 = Increment(x=w712) -> (x+1=w719:i32)
          n292 = Greater Or Equal?(x=w719, y=25) -> (x >= y?=w711:bool)
          n293 = call-poly <vilib>:"PID.vi"("PID gains"="PID gains 47", "process variable"=w714, "setpoint"=-70.0) -> ("output"=w706:dbl)  [unwired: 7 in, 1 out]
          "to motor 51" <- w706
          n294 = call-poly <vilib>:"WPI_RobotDriveHolonomicDrive.vi"("Rotation"=w706, "Y"=w710, "X"=w709, "RobotDriveDevRef"=w707) -> ("RobotDriveDevRef"=w708:T7)  [unwired: 5 in, 2 out]
          n295 = call-poly <vilib>:"NT Write Value.vi"("Numeric"=w713, "Name"="Gyro") -> ()  [unwired: 9 in, 1 out]
          n296 = Wait (ms)(milliseconds to wait=u32 20) -> ()  [unwired: 1 out]
        }
        n297 = while {
          tunnel: [w693] -> w606
          tunnel: w605 -> [w692]
          tunnel: w609 -> [w691]
          tunnel: [w691] -> w610
          i -> [w697]
          stop <- w696 stop-if-true
          w695 = -0.3  # Y
          w694 = 0.0  # X
          # "Drive Forward"
          n298 = call "SPI Gyro.vi"() -> ("Angle"=w698:dbl, "Raw"=w690:dbl)  [unwired: 9 in, 1 out]
          "Gauge 53" <- w690
          "Gryo angle 53" <- w690
          n299 = Increment(x=w697) -> (x+1=w703:i32)
          n300 = Greater Or Equal?(x=w703, y=5) -> (x >= y?=w696:bool)
          n301 = call-poly <vilib>:"PID.vi"("PID gains"="PID gains 46", "process variable"=w690, "setpoint"=-70.0) -> ("output"=w689:dbl)  [unwired: 7 in, 1 out]
          "to motor 50" <- w689
          n302 = call-poly <vilib>:"WPI_RobotDriveHolonomicDrive.vi"("Rotation"=w689, "Gyro Angle"=w690, "Y"=w695, "X"=w694, "RobotDriveDevRef"=w692) -> ("RobotDriveDevRef"=w693:T7)  [unwired: 4 in, 2 out]
          n303 = call-poly <vilib>:"NT Write Value.vi"("Numeric"=w698, "Name"="Gyro") -> ()  [unwired: 9 in, 1 out]
          n304 = Wait (ms)(milliseconds to wait=u32 20) -> ()  [unwired: 1 out]
        }
        n305 = while {
          tunnel: [w676] -> w612
          tunnel: w606 -> [w675]
          tunnel: w610 -> [w673]
          tunnel: [w672] -> w611
          i -> [w680]
          stop <- w679 stop-if-true
          w678 = 0.0  # Y
          w677 = 0.0  # X
          # "Place Gear"
          n306 = call "SPI Gyro.vi"() -> ("Angle"=w681:dbl, "Raw"=w682:dbl)  [unwired: 9 in, 1 out]
          "Gauge 52" <- w682
          "Gryo angle 52" <- w682
          n307 = Increment(x=w680) -> (x+1=w687:i32)
          n308 = Greater Or Equal?(x=w687, y=25) -> (x >= y?=w679:bool)
          n309 = call-poly <vilib>:"PID.vi"("PID gains"="PID gains 45", "process variable"=w682, "setpoint"=-70.0) -> ("output"=w671:dbl)  [unwired: 7 in, 1 out]
          "to motor 49" <- w671
          n310 = call-poly <vilib>:"WPI_SolenoidSet.vi"("Value"=WPI_SolenoidValue."Forward", "SolenoidDevRef"=w673) -> ("SolenoidDevRef"=w672:T5)  [unwired: 8 in, 1 out]
          n311 = call-poly <vilib>:"WPI_RobotDriveHolonomicDrive.vi"("Rotation"=w671, "Y"=w678, "X"=w677, "RobotDriveDevRef"=w675) -> ("RobotDriveDevRef"=w676:T7)  [unwired: 5 in, 2 out]
          n312 = call-poly <vilib>:"NT Write Value.vi"("Numeric"=w681, "Name"="Gyro") -> ()  [unwired: 9 in, 1 out]
          n313 = Wait (ms)(milliseconds to wait=u32 20) -> ()  [unwired: 1 out]
        }
        n314 = while {
          tunnel: [w659] -> w614
          tunnel: w612 -> [w658]
          tunnel: w611 -> [w656]
          tunnel: [w654] -> w613
          i -> [w663]
          stop <- w662 stop-if-true
          w661 = -0.3  # Y
          w660 = 0.0  # X
          # "Back Away and turn around"
          n315 = call "SPI Gyro.vi"() -> ("Angle"=w664:dbl, "Raw"=w653:dbl)  [unwired: 9 in, 1 out]
          "Gauge 51" <- w653
          "Gryo angle 51" <- w653
          n316 = Increment(x=w663) -> (x+1=w669:i32)
          n317 = Greater Or Equal?(x=w669, y=100) -> (x >= y?=w662:bool)
          n318 = call-poly <vilib>:"PID.vi"("PID gains"="PID gains 44", "process variable"=w653, "setpoint"=165.0) -> ("output"=w655:dbl)  [unwired: 7 in, 1 out]
          "to motor 48" <- w655
          n319 = call-poly <vilib>:"WPI_RobotDriveHolonomicDrive.vi"("Rotation"=w655, "Gyro Angle"=w653, "Y"=w661, "X"=w660, "RobotDriveDevRef"=w658) -> ("RobotDriveDevRef"=w659:T7)  [unwired: 4 in, 2 out]
          n320 = call-poly <vilib>:"WPI_SolenoidSet.vi"("Value"=WPI_SolenoidValue."Reverse", "SolenoidDevRef"=w656) -> ("SolenoidDevRef"=w654:T5)  [unwired: 8 in, 1 out]
          n321 = call-poly <vilib>:"NT Write Value.vi"("Numeric"=w664, "Name"="Gyro") -> ()  [unwired: 9 in, 1 out]
          n322 = Wait (ms)(milliseconds to wait=u32 20) -> ()  [unwired: 1 out]
        }
        n323 = while {
          tunnel: [w640] -> w615
          tunnel: w614 -> [w639]
          tunnel: w613 -> [w637]
          tunnel: [w634] -> w616
          i -> [w644]
          stop <- w643 stop-if-true
          w642 = -0.3  # Y
          w641 = 0.0  # X
          # "Drive to Key"
          n324 = call "SPI Gyro.vi"() -> ("Angle"=w645:dbl, "Raw"=w646:dbl)  [unwired: 9 in, 1 out]
          "Gauge 50" <- w646
          "Gryo angle 50" <- w646
          n325 = Increment(x=w644) -> (x+1=w651:i32)
          n326 = Greater Or Equal?(x=w651, y=100) -> (x >= y?=w643:bool)
          n327 = call-poly <vilib>:"PID.vi"("PID gains"="PID gains 43", "process variable"=w646, "setpoint"=0.0) -> ("output"=→"to motor 47":dbl)  [unwired: 7 in, 1 out]
          n328 = call-poly <vilib>:"WPI_RobotDriveHolonomicDrive.vi"("Rotation"=0.0, "Y"=w642, "X"=w641, "RobotDriveDevRef"=w639) -> ("RobotDriveDevRef"=w640:T7)  [unwired: 5 in, 2 out]
          n329 = call-poly <vilib>:"WPI_SolenoidSet.vi"("Value"=WPI_SolenoidValue."Off", "SolenoidDevRef"=w637) -> ("SolenoidDevRef"=w634:T5)  [unwired: 8 in, 1 out]
          n330 = call-poly <vilib>:"NT Write Value.vi"("Numeric"=w645, "Name"="Gyro") -> ()  [unwired: 9 in, 1 out]
          n331 = Wait (ms)(milliseconds to wait=u32 20) -> ()  [unwired: 1 out]
        }
        n332 = while {
          tunnel: [w622] -> _
          tunnel: w615 -> [w621]
          tunnel: [w618] -> _
          tunnel: w616 -> [w618]
          i -> [w626]
          stop <- w625 stop-if-true
          w624 = 0.0  # Y
          w623 = 0.0  # X
          # "Stop and shoot"
          n333 = call "SPI Gyro.vi"() -> ("Angle"=w627:dbl, "Raw"=w617:dbl)  [unwired: 9 in, 1 out]
          "Gauge 49" <- w617
          "Gryo angle 49" <- w617
          n334 = Increment(x=w626) -> (x+1=w632:i32)
          n335 = Greater Or Equal?(x=w632, y=100) -> (x >= y?=w625:bool)
          n336 = call-poly <vilib>:"PID.vi"("PID gains"="PID gains 42", "process variable"=w617, "setpoint"=0.0) -> ("output"=→"to motor 46":dbl)  [unwired: 7 in, 1 out]
          n337 = call-poly <vilib>:"WPI_RobotDriveHolonomicDrive.vi"("Rotation"=0.0, "Gyro Angle"=w617, "Y"=w624, "X"=w623, "RobotDriveDevRef"=w621) -> ("RobotDriveDevRef"=w622:T7)  [unwired: 4 in, 2 out]
          n338 = call-poly <vilib>:"NT Write Value.vi"("Numeric"=w627, "Name"="Gyro") -> ()  [unwired: 9 in, 1 out]
          n339 = Wait (ms)(milliseconds to wait=u32 20) -> ()  [unwired: 1 out]
        }
        n340 = Increment(x=w597) -> (x+1=w599:i32)
        n341 = Greater Or Equal?(x=w599, y=1) -> (x >= y?=w598:bool)
      }
    }
    frame "Drive strait" {
      n342 = while {
        tunnel: w745 -> [w752]
        i -> [w748]
        stop <- w749 stop-if-true
        n343 = while {
          tunnel: w752 -> [w783]
          tunnel: [w783] -> w747
          i -> [w785]
          stop <- w784 stop-if-true
          w786 = TRUE  # Reset
          n344 = Increment(x=w785) -> (x+1=w789:i32)
          n345 = call "SPI Gyro.vi"("Reset"=w786) -> ()  [unwired: 8 in, 3 out]
          n346 = Greater Or Equal?(x=w789, y=25) -> (x >= y?=w784:bool)
          n347 = Wait (ms)(milliseconds to wait=u32 20) -> ()  [unwired: 1 out]
        }
        n348 = while {
          tunnel: w747 -> [w769]
          tunnel: [w768] -> w746
          i -> [w774]
          stop <- w773 stop-if-true
          w772 = 0.3  # Y
          w771 = 0.0  # X
          n349 = call "SPI Gyro.vi"() -> ("Angle"=w775:dbl, "Raw"=w776:dbl)  [unwired: 9 in, 1 out]
          "Gauge 26" <- w776
          "Gryo angle 26" <- w776
          n350 = Increment(x=w774) -> (x+1=w781:i32)
          n351 = Greater Or Equal?(x=w781, y=125) -> (x >= y?=w773:bool)
          n352 = call-poly <vilib>:"PID.vi"("PID gains"="PID gains 19", "process variable"=w776, "setpoint"=0.0) -> ("output"=w770:dbl)  [unwired: 7 in, 1 out]
          "to motor 23" <- w770
          n353 = call-poly <vilib>:"WPI_RobotDriveHolonomicDrive.vi"("Rotation"=w770, "Y"=w772, "X"=w771, "RobotDriveDevRef"=w769) -> ("RobotDriveDevRef"=w768:T7)  [unwired: 5 in, 2 out]
          n354 = call-poly <vilib>:"NT Write Value.vi"("Numeric"=w775, "Name"="Gyro") -> ()  [unwired: 9 in, 1 out]
          n355 = Wait (ms)(milliseconds to wait=u32 20) -> ()  [unwired: 1 out]
        }
        n356 = while {
          i -> [w791]
          stop <- w790 stop-if-true
          (unwired) 0.3  # Y
          (unwired) 0.0  # X
          n357 = call "SPI Gyro.vi"() -> ("Angle"=w792:dbl, "Raw"=w793:dbl)  [unwired: 9 in, 1 out]
          "Gauge 19" <- w793
          "Gryo angle 19" <- w793
          n358 = Increment(x=w791) -> (x+1=w798:i32)
          n359 = Greater Or Equal?(x=w798, y=125) -> (x >= y?=w790:bool)
          n360 = call-poly <vilib>:"PID.vi"("PID gains"="PID gains 16", "process variable"=w793, "setpoint"=0.0) -> ()  [unwired: 7 in, 2 out]
          n361 = call-poly <vilib>:"NT Write Value.vi"("Numeric"=w792, "Name"="Gyro") -> ()  [unwired: 9 in, 1 out]
          n362 = Wait (ms)(milliseconds to wait=u32 20) -> ()  [unwired: 1 out]
        }
        n363 = while {
          tunnel: [w754] -> _
          tunnel: w746 -> [w753]
          i -> [w756]
          stop <- w755 stop-if-true
          w763 = 0.0  # Y
          w764 = 0.0  # X
          n364 = call "SPI Gyro.vi"() -> ("Angle"=w757:dbl, "Raw"=w758:dbl)  [unwired: 9 in, 1 out]
          "Gauge 28" <- w758
          "Gryo angle 28" <- w758
          n365 = Increment(x=w756) -> (x+1=w766:i32)
          n366 = Greater Or Equal?(x=w766, y=125) -> (x >= y?=w755:bool)
          n367 = call-poly <vilib>:"PID.vi"("PID gains"="PID gains 21", "process variable"=w758, "setpoint"=0.0) -> ("output"=w760:dbl)  [unwired: 7 in, 1 out]
          "to motor 25" <- w760
          n368 = call-poly <vilib>:"WPI_RobotDriveHolonomicDrive.vi"("Rotation"=w760, "Y"=w763, "X"=w764, "RobotDriveDevRef"=w753) -> ("RobotDriveDevRef"=w754:T7)  [unwired: 5 in, 2 out]
          n369 = call-poly <vilib>:"NT Write Value.vi"("Numeric"=w757, "Name"="Gyro") -> ()  [unwired: 9 in, 1 out]
          n370 = Wait (ms)(milliseconds to wait=u32 20) -> ()  [unwired: 1 out]
        }
        n371 = Increment(x=w748) -> (x+1=w750:i32)
        n372 = Greater Or Equal?(x=w750, y=4) -> (x >= y?=w749:bool)
      }
    }
    frame "Square" {
      n373 = while {
        tunnel: w800 -> [w808]
        i -> [w801]
        stop <- w802 stop-if-true
        n374 = while {
          tunnel: [w846] -> w809
          tunnel: w808 -> [w846]
          i -> [w842]
          stop <- w843 stop-if-true
          w840 = TRUE  # Reset
          n375 = Increment(x=w842) -> (x+1=w845:i32)
          n376 = call "SPI Gyro.vi"("Reset"=w840) -> ()  [unwired: 8 in, 3 out]
          n377 = Greater Or Equal?(x=w845, y=25) -> (x >= y?=w843:bool)
          n378 = Wait (ms)(milliseconds to wait=u32 20) -> ()  [unwired: 1 out]
        }
        n379 = while {
          tunnel: [w839] -> w807
          tunnel: w809 -> [w828]
          i -> [w837]
          stop <- w834 stop-if-true
          w832 = -0.3  # Y
          w833 = 0.0  # X
          n380 = call "SPI Gyro.vi"() -> ("Angle"=w825:dbl, "Raw"=w826:dbl)  [unwired: 9 in, 1 out]
          "Gauge 9" <- w826
          "Gryo angle 9" <- w826
          n381 = Increment(x=w837) -> (x+1=w836:i32)
          n382 = Greater Or Equal?(x=w836, y=125) -> (x >= y?=w834:bool)
          n383 = call-poly <vilib>:"PID.vi"("PID gains"="PID gains 6", "process variable"=w826, "setpoint"=0.0) -> ("output"=w829:dbl)  [unwired: 7 in, 1 out]
          "to motor 6" <- w829
          n384 = call-poly <vilib>:"WPI_RobotDriveHolonomicDrive.vi"("Rotation"=w829, "Y"=w832, "X"=w833, "RobotDriveDevRef"=w828) -> ("RobotDriveDevRef"=w839:T7)  [unwired: 5 in, 2 out]
          n385 = call-poly <vilib>:"NT Write Value.vi"("Numeric"=w825, "Name"="Gyro") -> ()  [unwired: 9 in, 1 out]
          n386 = Wait (ms)(milliseconds to wait=u32 20) -> ()  [unwired: 1 out]
        }
        n387 = while {
          tunnel: [w824] -> w806
          tunnel: w807 -> [w813]
          i -> [w822]
          stop <- w819 stop-if-true
          w817 = 0.0  # Y
          w818 = 0.3  # X
          n388 = call "SPI Gyro.vi"() -> ("Angle"=w810:dbl, "Raw"=w811:dbl)  [unwired: 9 in, 1 out]
          "Gauge 10" <- w811
          "Gryo angle 10" <- w811
          n389 = Increment(x=w822) -> (x+1=w821:i32)
          n390 = Greater Or Equal?(x=w821, y=125) -> (x >= y?=w819:bool)
          n391 = call-poly <vilib>:"PID.vi"("PID gains"="PID gains 7", "process variable"=w811, "setpoint"=0.0) -> ("output"=w814:dbl)  [unwired: 7 in, 1 out]
          "to motor 7" <- w814
          n392 = call-poly <vilib>:"WPI_RobotDriveHolonomicDrive.vi"("Rotation"=w814, "Y"=w817, "X"=w818, "RobotDriveDevRef"=w813) -> ("RobotDriveDevRef"=w824:T7)  [unwired: 5 in, 2 out]
          n393 = call-poly <vilib>:"NT Write Value.vi"("Numeric"=w810, "Name"="Gyro") -> ()  [unwired: 9 in, 1 out]
          n394 = Wait (ms)(milliseconds to wait=u32 20) -> ()  [unwired: 1 out]
        }
        n395 = while {
          tunnel: [w876] -> w805
          tunnel: w806 -> [w865]
          i -> [w874]
          stop <- w871 stop-if-true
          w869 = 0.3  # Y
          w870 = 0.0  # X
          n396 = call "SPI Gyro.vi"() -> ("Angle"=w862:dbl, "Raw"=w863:dbl)  [unwired: 9 in, 1 out]
          "Gauge 11" <- w863
          "Gryo angle 11" <- w863
          n397 = Increment(x=w874) -> (x+1=w873:i32)
          n398 = Greater Or Equal?(x=w873, y=125) -> (x >= y?=w871:bool)
          n399 = call-poly <vilib>:"PID.vi"("PID gains"="PID gains 8", "process variable"=w863, "setpoint"=0.0) -> ("output"=w866:dbl)  [unwired: 7 in, 1 out]
          "to motor 8" <- w866
          n400 = call-poly <vilib>:"WPI_RobotDriveHolonomicDrive.vi"("Rotation"=w866, "Y"=w869, "X"=w870, "RobotDriveDevRef"=w865) -> ("RobotDriveDevRef"=w876:T7)  [unwired: 5 in, 2 out]
          n401 = call-poly <vilib>:"NT Write Value.vi"("Numeric"=w862, "Name"="Gyro") -> ()  [unwired: 9 in, 1 out]
          n402 = Wait (ms)(milliseconds to wait=u32 20) -> ()  [unwired: 1 out]
        }
        n403 = while {
          tunnel: [w861] -> _
          tunnel: w805 -> [w850]
          i -> [w859]
          stop <- w856 stop-if-true
          w854 = 0.0  # Y
          w855 = -0.3  # X
          n404 = call "SPI Gyro.vi"() -> ("Angle"=w847:dbl, "Raw"=w848:dbl)  [unwired: 9 in, 1 out]
          "Gauge 15" <- w848
          "Gryo angle 15" <- w848
          n405 = Increment(x=w859) -> (x+1=w858:i32)
          n406 = Greater Or Equal?(x=w858, y=125) -> (x >= y?=w856:bool)
          n407 = call-poly <vilib>:"PID.vi"("PID gains"="PID gains 12", "process variable"=w848, "setpoint"=0.0) -> ("output"=w851:dbl)  [unwired: 7 in, 1 out]
          "to motor 12" <- w851
          n408 = call-poly <vilib>:"WPI_RobotDriveHolonomicDrive.vi"("Rotation"=w851, "Y"=w854, "X"=w855, "RobotDriveDevRef"=w850) -> ("RobotDriveDevRef"=w861:T7)  [unwired: 5 in, 2 out]
          n409 = call-poly <vilib>:"NT Write Value.vi"("Numeric"=w847, "Name"="Gyro") -> ()  [unwired: 9 in, 1 out]
          n410 = Wait (ms)(milliseconds to wait=u32 20) -> ()  [unwired: 1 out]
        }
        n411 = Increment(x=w801) -> (x+1=w803:i32)
        n412 = Greater Or Equal?(x=w803, y=4) -> (x >= y?=w802:bool)
      }
    }
  }
  n413 = call <vilib>:"WPI_DriverStationGet Alliance Info.vi"() -> ()  [unwired: 12 out]
  n414 = while {
    stop <- FALSE stop-if-true
    n415 = call <vilib>:"WPI_DriverStationReport Robot Code State.vi"("Autonomous"=TRUE) -> ()  [unwired: 10 in, 1 out]
    n416 = Wait (ms)(milliseconds to wait=u32 20) -> ()  [unwired: 1 out]
  }
